vi "Part Config.vi"(0 "Loaded Config":T2={"DAQ Settings"={"Trigger Type"=enum."Manual", "Trigger Samples"=0, "Pretrigger Samples"=0, "Trigger Interval"=0.0, "Time Units"=FALSE, "Auto Save"=FALSE, "Sample Rate"=7.0, "Select Analog"=FALSE, "Trigger Value"=0.0, "Trigger Stop Method"=enum."Use Samples Value to Stop Trigger", "Rate Sec/Min"=FALSE, "Save Mode"=enum."Single File", "File Size Limit"=0.0, "Log File Type"=enum."Basic", "Trigger Data Index"=0}, "Channels"=[], "Header"={"TA Number"="", "Test Name"="", "Serial Number"="", "Technician"=""}, "Graph Settings"={"Graph Labels"=[], [], [], [], [], [], [], [], [], [], [], [], [], "Graph Toggles"=[], "Axis Toggles"=[], "Graph Range"=enum."1"}, "Test Limits"=[], "All Type Info"=[], "Save Mode"=enum."Single File"} {"DAQ Settings"."Trigger Interval" min=0.0; "DAQ Settings"."Pretrigger Samples" min=0; "DAQ Settings"."Trigger Samples" min=0}) -> (4 "Config Out":T2={"DAQ Settings"={"Trigger Type"=enum."Manual", "Trigger Samples"=0, "Pretrigger Samples"=0, "Trigger Interval"=0.0, "Time Units"=FALSE, "Auto Save"=FALSE, "Sample Rate"=7.0, "Select Analog"=FALSE, "Trigger Value"=0.0, "Trigger Stop Method"=enum."Use Samples Value to Stop Trigger", "Rate Sec/Min"=FALSE, "Save Mode"=enum."Single File", "File Size Limit"=0.0, "Log File Type"=enum."Basic", "Trigger Data Index"=0}, "Channels"=[], "Header"={"TA Number"="", "Test Name"="", "Serial Number"="", "Technician"=""}, "Graph Settings"={"Graph Labels"=[], [], [], [], [], [], [], [], [], [], [], [], [], "Graph Toggles"=[], "Axis Toggles"=[], "Graph Range"=enum."1"}, "Test Limits"=[], "All Type Info"=[], "Save Mode"=enum."Single File"} {"DAQ Settings"."Trigger Interval" min=0.0; "DAQ Settings"."Pretrigger Samples" min=0; "DAQ Settings"."Trigger Samples" min=0}, 8 "Changes?":bool)   [LabVIEW 2019]
uses:
  Type Defs and Controls/Sensor Config.ctl
  Type Defs and Controls/DAQ Settings.ctl
  Type Defs and Controls/Trigger Stop Method.ctl
  Type Defs and Controls/Log File Type.ctl
  Type Defs and Controls/Channel Config.ctl
  Type Defs and Controls/Header.ctl
  Type Defs and Controls/Graph Settings Type Def.ctl
  Type Defs and Controls/Test Limits.ctl
  Type Defs and Controls/All Part Info.ctl
  Type Defs and Controls/Part Info.ctl
panel:
  in  "Rename":bool
  out "Total Channels":string
  in  "Delete Type":bool
  in  "Add New Type":bool
  in  "Type":u16(ring) items=["<NO SELECTION >", "New Type"]
  in  "Tab Control":enum32{"Main", "Limits"}(tab)
  in  "Part Numbers":cluster{"Part Number":string, "Acquire":bool}[](array[cluster])
  in  "Signals  Names":T1(array[cluster])
  in  "# Signals":u16=1 min=1 max=32 step=1
  in  "# Parts":u16=1 min=1 max=32 step=1
  in  "Signal Style":enum16{"Steady State", "Cyclic"}(ring)
  out "Current Limit Selection:":string
  in  "RMS Minimum":dbl format="%.3f "
  in  "RMS Maximum":dbl format="%.3f "
  in  "Enable Limits":bool
  in  "Pk-Pk Minimum":dbl format="%.3f "
  in  "Pk-Pk Maximum":dbl format="%.3f "
  in  "Enable Limits":bool
  in  "EU Low State Min":dbl format="%.3f "
  in  "EU Low State Max":dbl format="%.3f "
  in  "EU High State Min":dbl caption="EU Minimum" format="%.3f "
  in  "EU High State Max":dbl caption="EU Maximum" format="%.3f "
  in  "Freq Minimum":dbl format="%.1f Hz"
  in  "Freq Maximum":dbl format="%.1f Hz"
  in  "Enable Limits":bool
  in  "Cancel":bool
  in  "OK":bool
  # "All Signals that have matching High and Low Limits\nwill not be in Functional data file."
  # "RMS Limits"
  # "EU Limits Type"
  # "Pk-Pk Limits"
  # "Frequency Limits"
  # "All Signals that have matching High and Low Limits will not be in Functional data file."
  # "EGU"
  # "EGU"
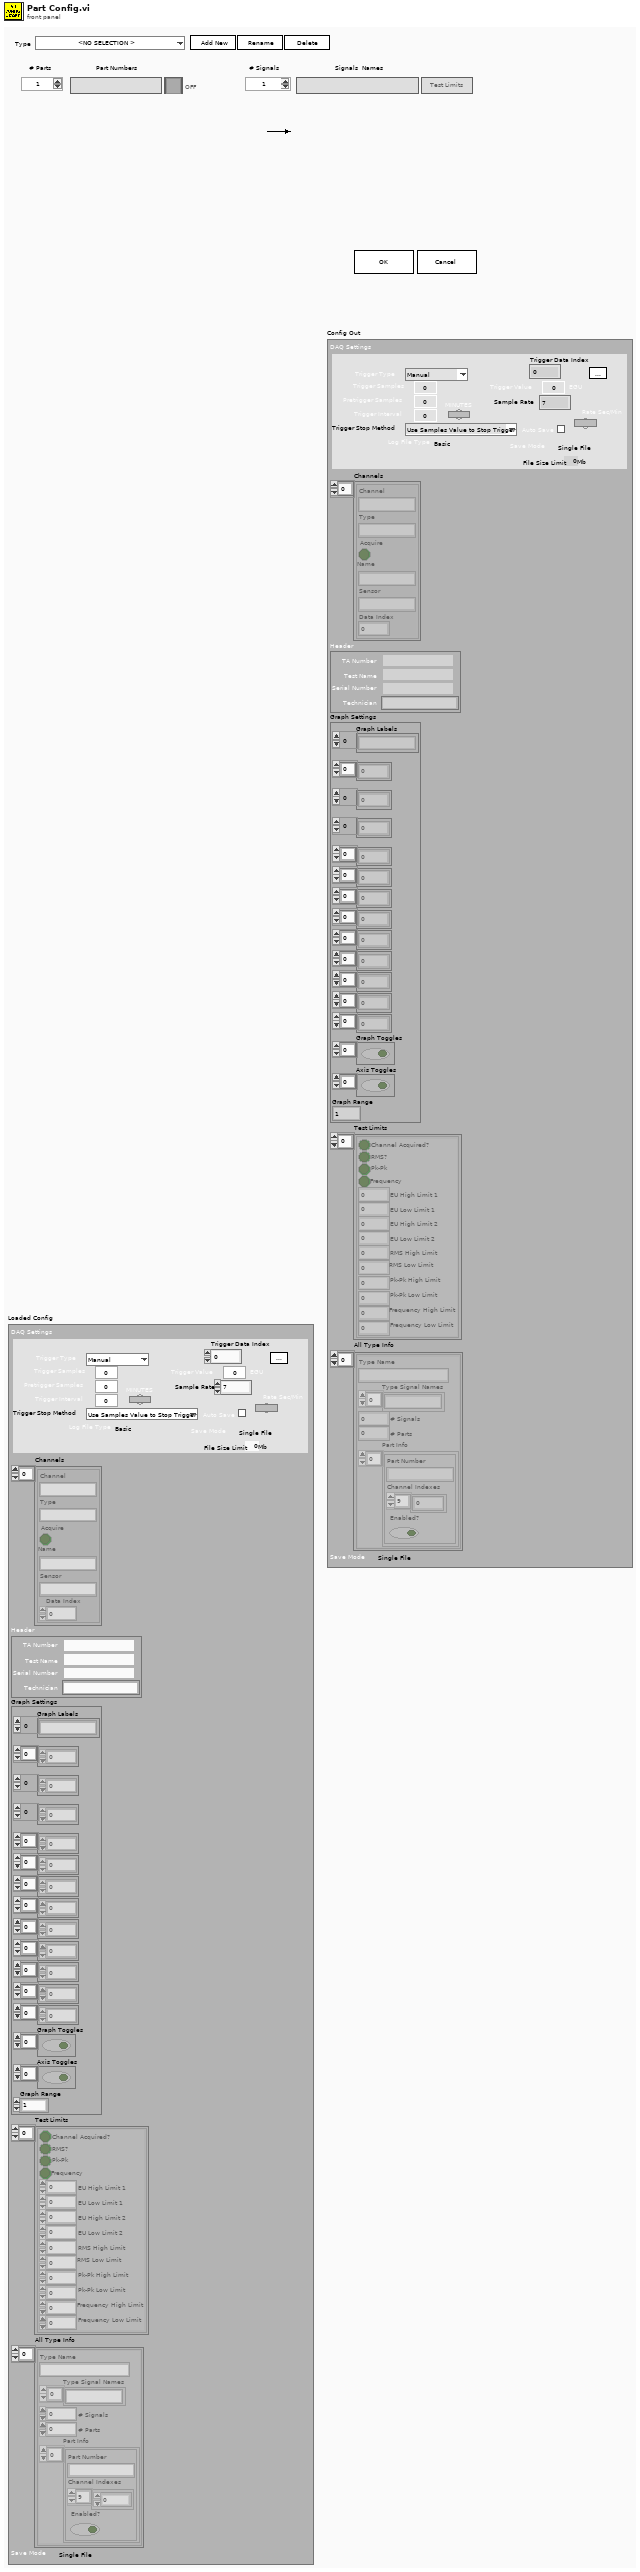
[diagram p1: front panel]
types:
  T1 = cluster{"Signal Names":string, "Test Limits":bool}[]
  T2 = typedef "Sensor Config.ctl" = cluster{"DAQ Settings":T3, "Channels":T6[], "Header":T7, "Graph Settings":T8, "Test Limits":T9[], "All Type Info":T10, "Save Mode":enum16{"Single File", "Segmented Files", "New File at Midnight"}}
  T3 = typedef "DAQ Settings.ctl" = cluster{"Trigger Type":enum16{"Manual", "Timed", "Analog Rising", "Analog Falling"}, "Trigger Samples":i32, "Pretrigger Samples":i32, "Trigger Interval":dbl, "Time Units":bool, "Auto Save":bool, "Sample Rate":dbl, "Select Analog":bool, "Trigger Value":dbl, "Trigger Stop Method":T4, "Rate Sec/Min":bool, "Save Mode":enum16{"Single File", "Segmented Files", "New File at Midnight"}, "File Size Limit":dbl, "Log File Type":T5, "Trigger Data Index":u32}
  T4 = typedef "Trigger Stop Method.ctl" = enum16{"Use Samples Value to Stop Trigger", "Use Threshold to Stop Trigger"}
  T5 = typedef "Log File Type.ctl" = enum16{"Basic", "RTS"}
  T6 = typedef "Channel Config.ctl" = cluster{"Channel":string, "Type":string, "Acquire":bool, "Name":string, "Sensor":string, "Data Index":u32}
  T7 = typedef "Header.ctl" = cluster{"TA Number":string, "Test Name":string, "Serial Number":string, "Technician":string}
  T8 = typedef "Graph Settings Type Def.ctl" = cluster{"Graph Labels":string[], u8[], i16[], u32[], u8[], u8[], u8[], u32[], u8[], u8[], u8[], dbl[], dbl[], "Graph Toggles":bool[], "Axis Toggles":bool[], "Graph Range":enum16{"1", "2", "3", "4", "5", "10", "15", "30", "60"}}
  T9 = typedef "Test Limits.ctl" = cluster{"Channel Acquired?":bool, "RMS?":bool, "Pk-Pk":bool, "Frequency":bool, "EU High Limit 1":dbl, "EU Low Limit 1":dbl, "EU High Limit 2":dbl, "EU Low Limit 2":dbl, "RMS High Limit":dbl, "RMS Low Limit":dbl, "Pk-Pk High Limit ":dbl, "Pk-Pk Low Limit":dbl, "Frequency High Limit":dbl, "Frequency Low Limit":dbl}
  T10 = typedef "All Part Info.ctl" = cluster{"Type Name":string, "Type Signal Names":string[], "# Signals":i32, "# Parts":i32, "Part Info":T11[]}[]
  T11 = typedef "Part Info.ctl" = cluster{"Part Number":string, "Channel Indexes":u16[], "Enabled?":bool}
  T12 = cluster{"Loaded Config":T2, "Modified Config":T2, "Test Limit Index":i32, "Type Index":i32, "All Test Limits":cluster{T9[]}[], "All Type Info":T10, "Last Type Index":i32, "Signal Style Index":i32, "Last Signal Style Index":i32}
  T13 = enum8{"Enabled", "Disabled", "Disabled and Grayed Out"}
  T14 = cluster{"Type Name":string, "Type Signal Names":string[], "# Signals":i32, "# Parts":i32, "Type Info":T11[]}
  T15 = cluster{"Type Name":string, "Type Signal Names":string[], "# Signals":i32, "# Parts":i32, "Part Info":T11[]}
  T16 = cluster{"Type Name":string, "Type Signal Names":string[], "Signals":i32, "# Parts":i32, "Type Info":T11[]}[]
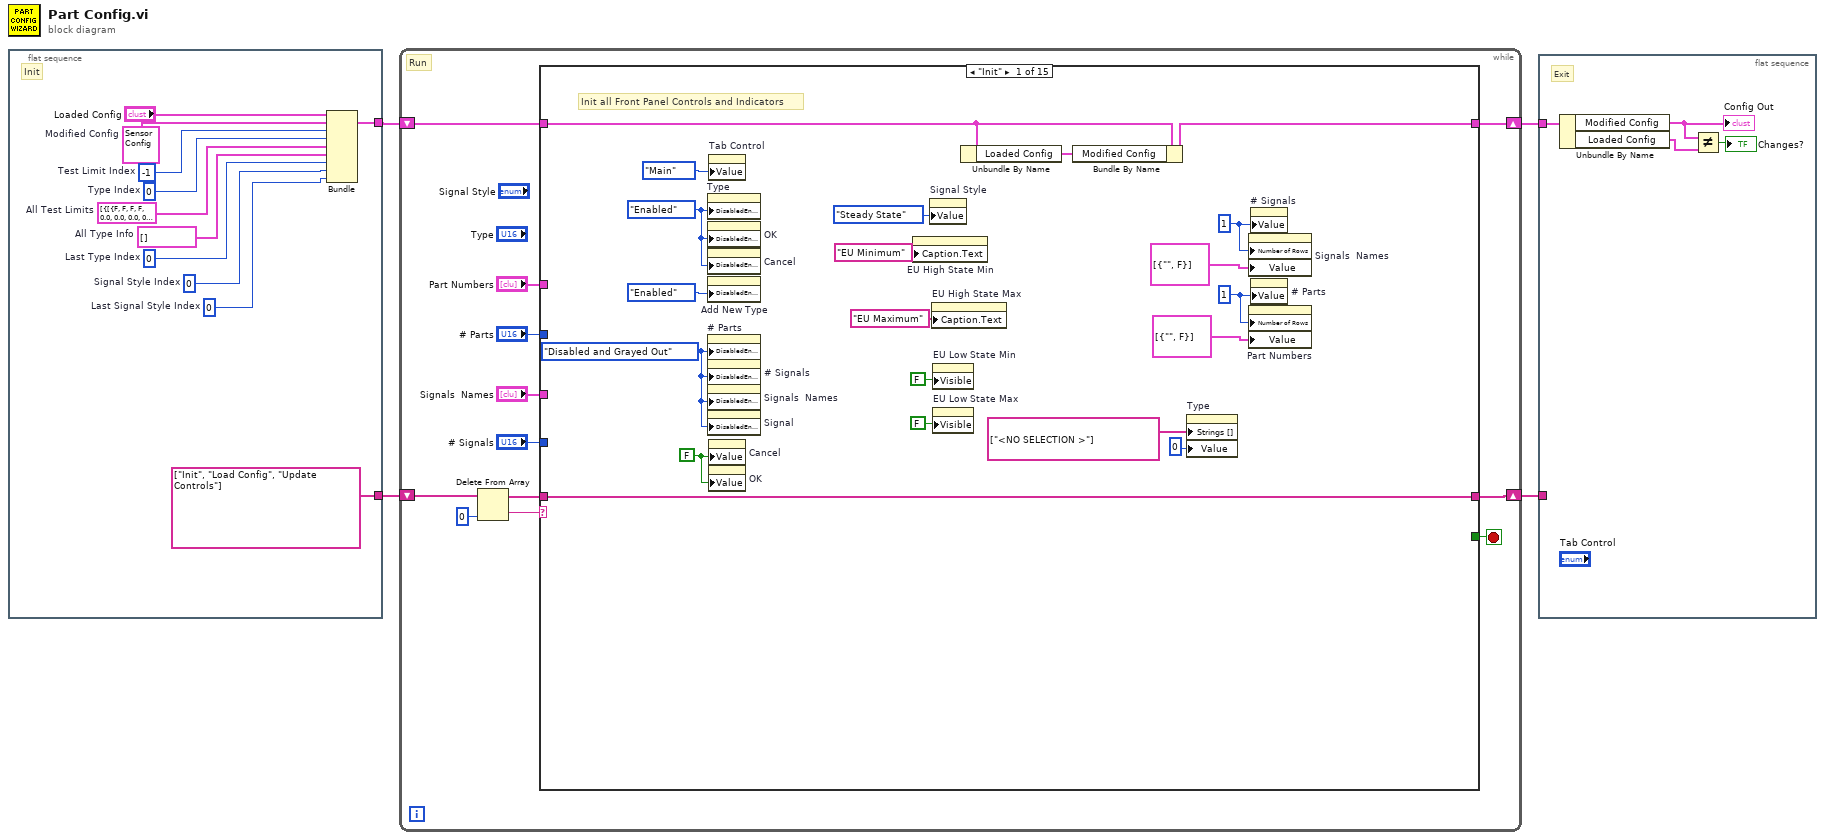
[diagram p0: block diagram]
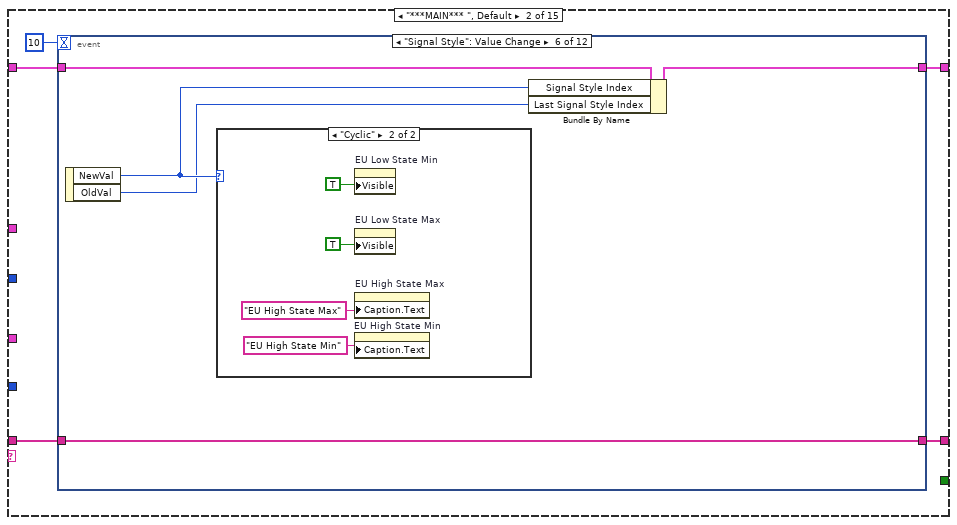
[diagram p2: hidden frame]
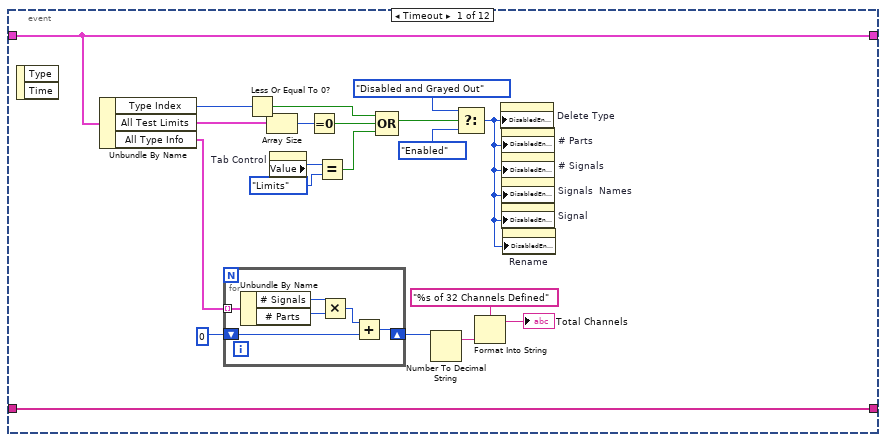
[diagram p3: hidden frame]
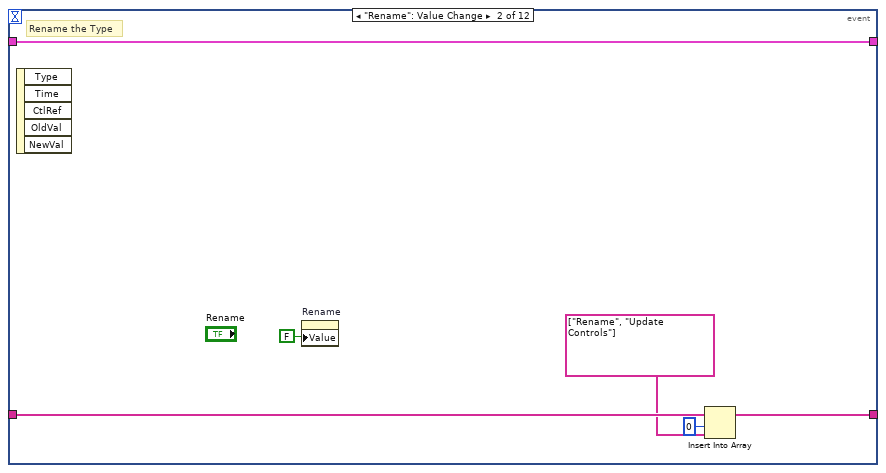
[diagram p4: hidden frame]
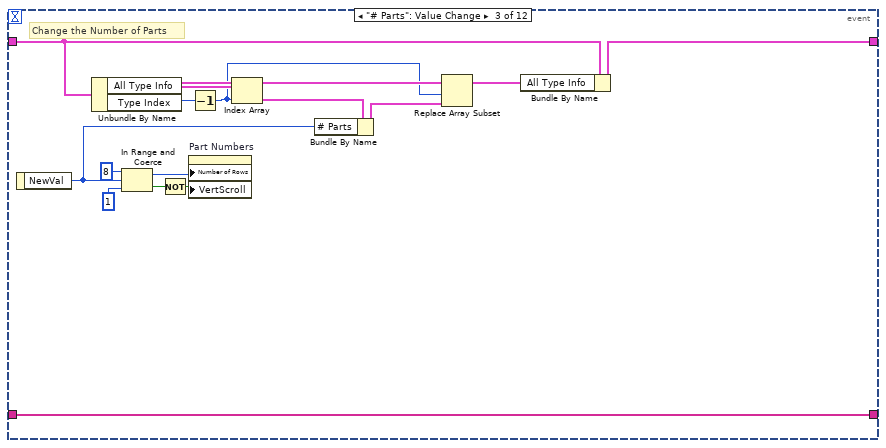
[diagram p5: hidden frame]
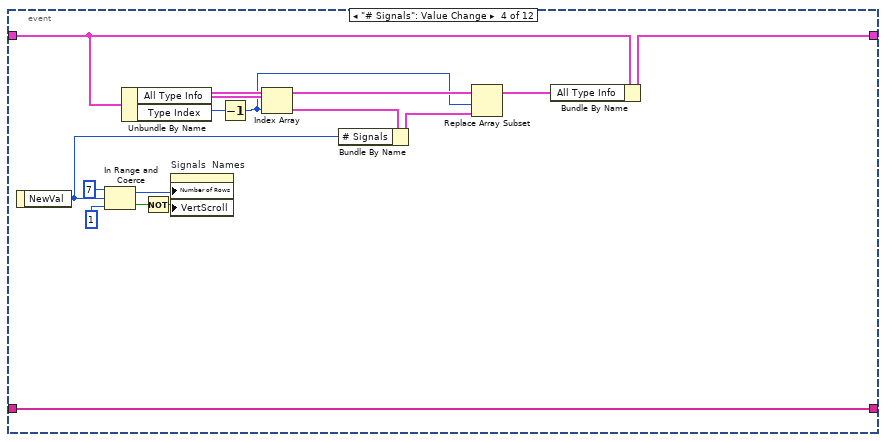
[diagram p6: hidden frame]
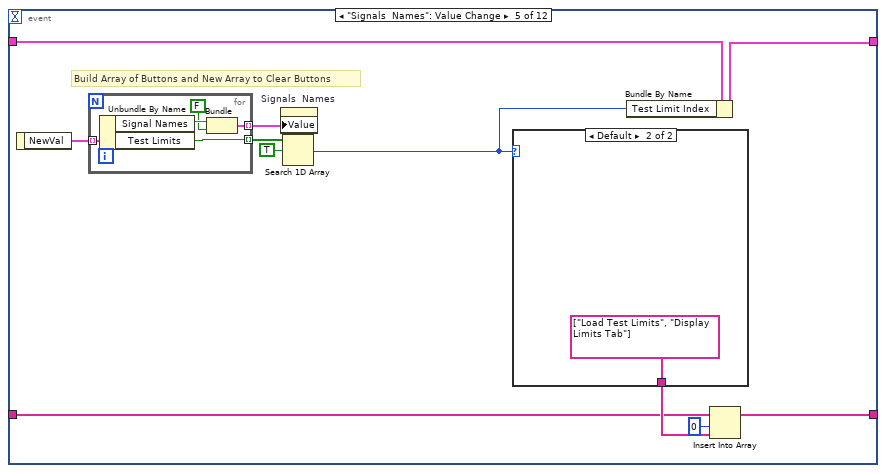
[diagram p7: hidden frame]
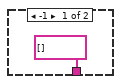
[diagram p8: hidden frame]
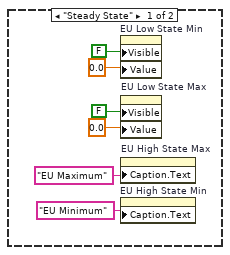
[diagram p9: hidden frame]
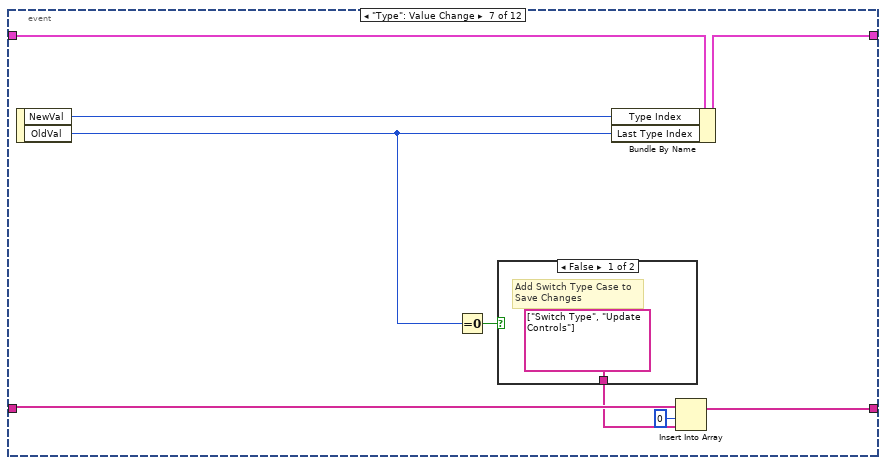
[diagram p10: hidden frame]
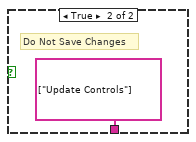
[diagram p11: hidden frame]
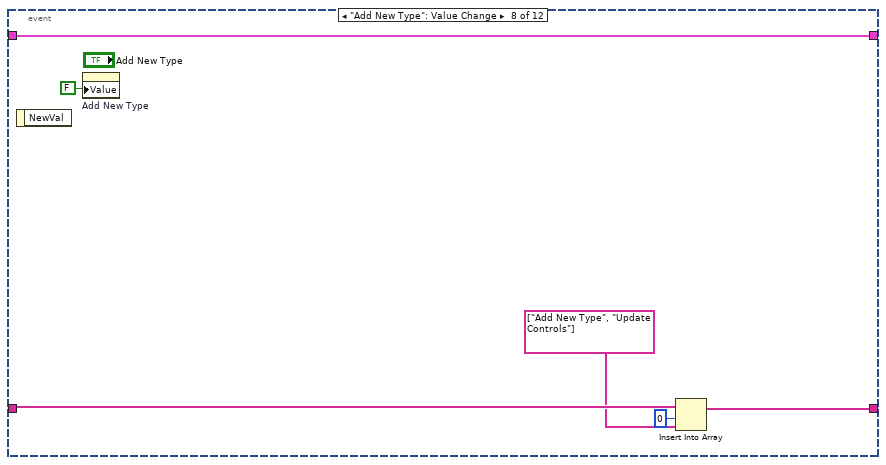
[diagram p12: hidden frame]
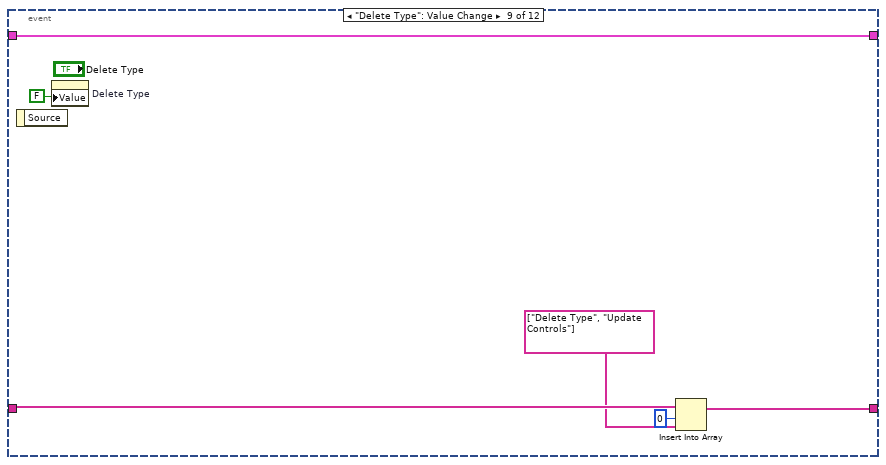
[diagram p13: hidden frame]
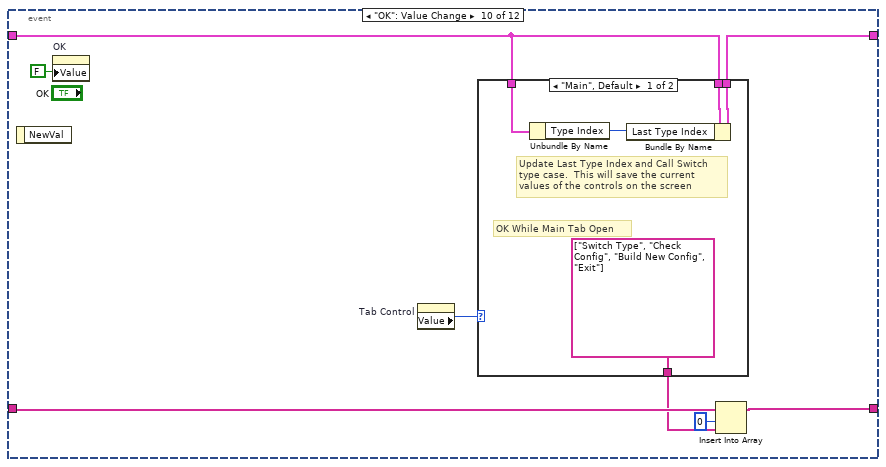
[diagram p14: hidden frame]
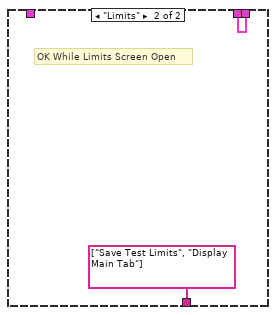
[diagram p15: hidden frame]
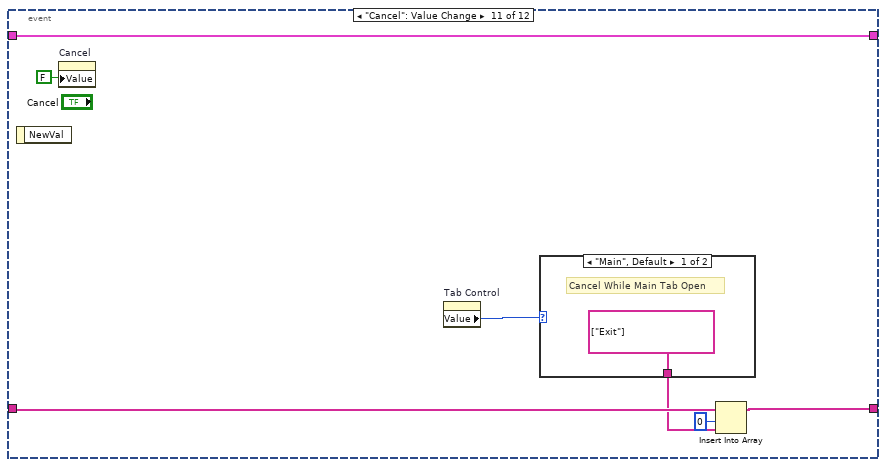
[diagram p16: hidden frame]
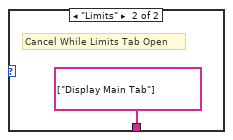
[diagram p17: hidden frame]
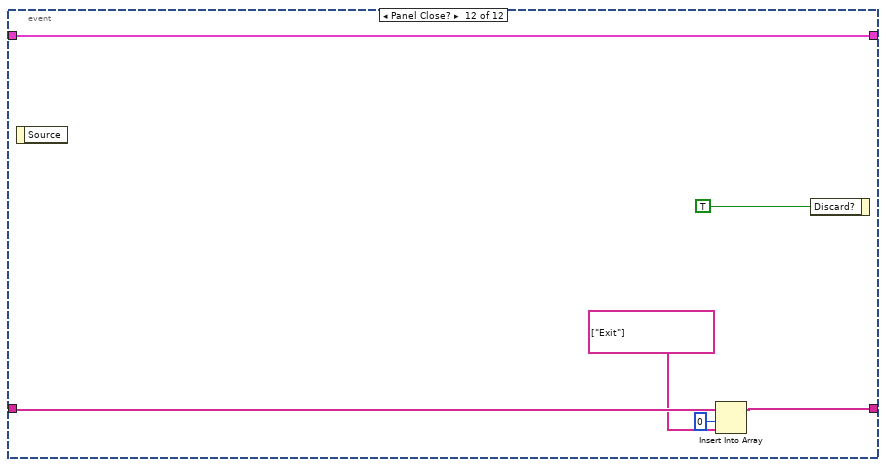
[diagram p18: hidden frame]
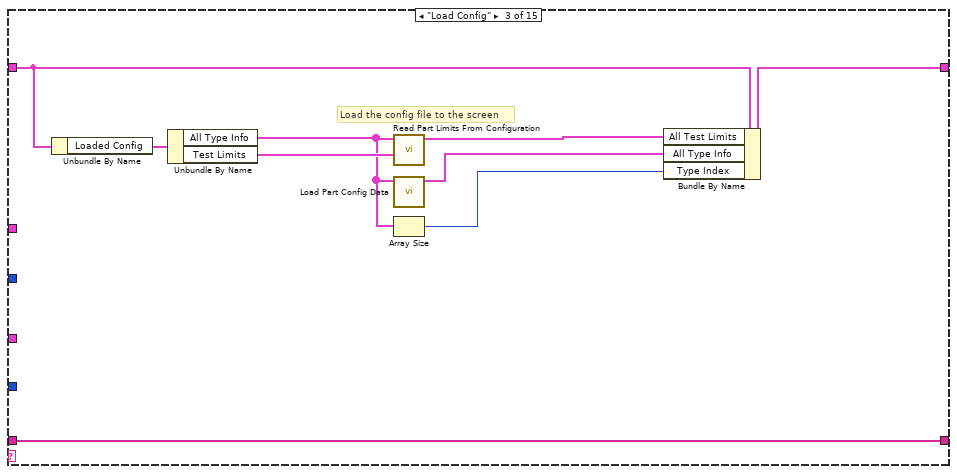
[diagram p19: hidden frame]
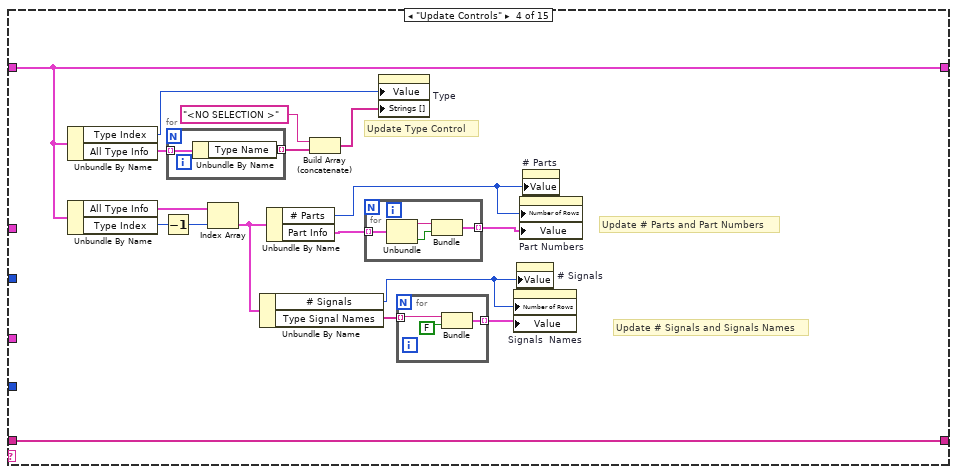
[diagram p20: hidden frame]
diagram:
  n1 = flat-sequence {
    tunnel: [string[] ["Init", "Load Config", "Update Controls"]] -> w4
    tunnel: [w14] -> w3
    frame #0 {
      w5 = 0  # Last Signal Style Index
      w6 = 0  # Signal Style Index
      w7 = 0  # Last Type Index
      w8 = T10 []  # All Type Info
      w9 = cluster{T9[]}[] [{[{"Channel Acquired?"=FALSE, "RMS?"=FALSE, "Pk-Pk"=FALSE, "Frequency"=FALSE, "EU High Limit 1"=0.0, "EU Low Limit 1"=0.0, "EU High Limit 2"=0.0, "EU Low Limit 2"=0.0, "RMS High Limit"=0.0, "RMS Low Limit"=0.0, "Pk-Pk High Limit "=0.0, "Pk-Pk Low Limit"=0.0, "Frequency High Limit"=0.0, "Frequency Low Limit"=0.0}]}, {[{"Channel Acquired?"=FALSE, "RMS?"=FALSE, "Pk-Pk"=FALSE, "Frequency"=FALSE, "EU High Limit 1"=0.0, "EU Low Limit 1"=0.0, "EU High Limit 2"=0.0, "EU Low Limit 2"=0.0, "RMS High Limit"=0.0, "RMS Low Limit"=0.0, "Pk-Pk High Limit "=0.0, "Pk-Pk Low Limit"=0.0, "Frequency High Limit"=0.0, "Frequency Low Limit"=0.0}]}, {[{"Channel Acquired?"=FALSE, "RMS?"=FALSE, "Pk-Pk"=FALSE, "Frequency"=FALSE, "EU High Limit 1"=0.0, "EU Low Limit 1"=0.0, "EU High Limit 2"=0.0, "EU Low Limit 2"=0.0, "RMS High Limit"=0.0, "RMS Low Limit"=0.0, "Pk-Pk High Limit "=0.0, "Pk-Pk Low Limit"=0.0, "Frequency High Limit"=0.0, "Frequency Low Limit"=0.0}]}, {[{"Channel Acquired?"=FALSE, "RMS?"=FALSE, "Pk-Pk"=FALSE, "Frequency"=FALSE, "EU High Limit 1"=0.0, "EU Low Limit 1"=0.0, "EU High Limit 2"=0.0, "EU Low Limit 2"=0.0, "RMS High Limit"=0.0, "RMS Low Limit"=0.0, "Pk-Pk High Limit "=0.0, "Pk-Pk Low Limit"=0.0, "Frequency High Limit"=0.0, "Frequency Low Limit"=0.0}]}, {[{"Channel Acquired?"=FALSE, "RMS?"=FALSE, "Pk-Pk"=FALSE, "Frequency"=FALSE, "EU High Limit 1"=0.0, "EU Low Limit 1"=0.0, "EU High Limit 2"=0.0, "EU Low Limit 2"=0.0, "RMS High Limit"=0.0, "RMS Low Limit"=0.0, "Pk-Pk High Limit "=0.0, "Pk-Pk Low Limit"=0.0, "Frequency High Limit"=0.0, "Frequency Low Limit"=0.0}]}, {[{"Channel Acquired?"=FALSE, "RMS?"=FALSE, "Pk-Pk"=FALSE, "Frequency"=FALSE, "EU High Limit 1"=0.0, "EU Low Limit 1"=0.0, "EU High Limit 2"=0.0, "EU Low Limit 2"=0.0, "RMS High Limit"=0.0, "RMS Low Limit"=0.0, "Pk-Pk High Limit "=0.0, "Pk-Pk Low Limit"=0.0, "Frequency High Limit"=0.0, "Frequency Low Limit"=0.0}]}, {[{"Channel Acquired?"=FALSE, "RMS?"=FALSE, "Pk-Pk"=FALSE, "Frequency"=FALSE, "EU High Limit 1"=0.0, "EU Low Limit 1"=0.0, "EU High Limit 2"=0.0, "EU Low Limit 2"=0.0, "RMS High Limit"=0.0, "RMS Low Limit"=0.0, "Pk-Pk High Limit "=0.0, "Pk-Pk Low Limit"=0.0, "Frequency High Limit"=0.0, "Frequency Low Limit"=0.0}]}, {[{"Channel Acquired?"=FALSE, "RMS?"=FALSE, "Pk-Pk"=FALSE, "Frequency"=FALSE, "EU High Limit 1"=0.0, "EU Low Limit 1"=0.0, "EU High Limit 2"=0.0, "EU Low Limit 2"=0.0, "RMS High Limit"=0.0, "RMS Low Limit"=0.0, "Pk-Pk High Limit "=0.0, "Pk-Pk Low Limit"=0.0, "Frequency High Limit"=0.0, "Frequency Low Limit"=0.0}]}, {[{"Channel Acquired?"=FALSE, "RMS?"=FALSE, "Pk-Pk"=FALSE, "Frequency"=FALSE, "EU High Limit 1"=0.0, "EU Low Limit 1"=0.0, "EU High Limit 2"=0.0, "EU Low Limit 2"=0.0, "RMS High Limit"=0.0, "RMS Low Limit"=0.0, "Pk-Pk High Limit "=0.0, "Pk-Pk Low Limit"=0.0, "Frequency High Limit"=0.0, "Frequency Low Limit"=0.0}]}, {[{"Channel Acquired?"=FALSE, "RMS?"=FALSE, "Pk-Pk"=FALSE, "Frequency"=FALSE, "EU High Limit 1"=0.0, "EU Low Limit 1"=0.0, "EU High Limit 2"=0.0, "EU Low Limit 2"=0.0, "RMS High Limit"=0.0, "RMS Low Limit"=0.0, "Pk-Pk High Limit "=0.0, "Pk-Pk Low Limit"=0.0, "Frequency High Limit"=0.0, "Frequency Low Limit"=0.0}]}, {[{"Channel Acquired?"=FALSE, "RMS?"=FALSE, "Pk-Pk"=FALSE, "Frequency"=FALSE, "EU High Limit 1"=0.0, "EU Low Limit 1"=0.0, "EU High Limit 2"=0.0, "EU Low Limit 2"=0.0, "RMS High Limit"=0.0, "RMS Low Limit"=0.0, "Pk-Pk High Limit "=0.0, "Pk-Pk Low Limit"=0.0, "Frequency High Limit"=0.0, "Frequency Low Limit"=0.0}]}, {[{"Channel Acquired?"=FALSE, "RMS?"=FALSE, "Pk-Pk"=FALSE, "Frequency"=FALSE, "EU High Limit 1"=0.0, "EU Low Limit 1"=0.0, "EU High Limit 2"=0.0, "EU Low Limit 2"=0.0, "RMS High Limit"=0.0, "RMS Low Limit"=0.0, "Pk-Pk High Limit "=0.0, "Pk-Pk Low Limit"=0.0, "Frequency High Limit"=0.0, "Frequency Low Limit"=0.0}]}, {[{"Channel Acquired?"=FALSE, "RMS?"=FALSE, "Pk-Pk"=FALSE, "Frequency"=FALSE, "EU High Limit 1"=0.0, "EU Low Limit 1"=0.0, "EU High Limit 2"=0.0, "EU Low Limit 2"=0.0, "RMS High Limit"=0.0, "RMS Low Limit"=0.0, "Pk-Pk High Limit "=0.0, "Pk-Pk Low Limit"=0.0, "Frequency High Limit"=0.0, "Frequency Low Limit"=0.0}]}, {[{"Channel Acquired?"=FALSE, "RMS?"=FALSE, "Pk-Pk"=FALSE, "Frequency"=FALSE, "EU High Limit 1"=0.0, "EU Low Limit 1"=0.0, "EU High Limit 2"=0.0, "EU Low Limit 2"=0.0, "RMS High Limit"=0.0, "RMS Low Limit"=0.0, "Pk-Pk High Limit "=0.0, "Pk-Pk Low Limit"=0.0, "Frequency High Limit"=0.0, "Frequency Low Limit"=0.0}]}, {[{"Channel Acquired?"=FALSE, "RMS?"=FALSE, "Pk-Pk"=FALSE, "Frequency"=FALSE, "EU High Limit 1"=0.0, "EU Low Limit 1"=0.0, "EU High Limit 2"=0.0, "EU Low Limit 2"=0.0, "RMS High Limit"=0.0, "RMS Low Limit"=0.0, "Pk-Pk High Limit "=0.0, "Pk-Pk Low Limit"=0.0, "Frequency High Limit"=0.0, "Frequency Low Limit"=0.0}]}, {[{"Channel Acquired?"=FALSE, "RMS?"=FALSE, "Pk-Pk"=FALSE, "Frequency"=FALSE, "EU High Limit 1"=0.0, "EU Low Limit 1"=0.0, "EU High Limit 2"=0.0, "EU Low Limit 2"=0.0, "RMS High Limit"=0.0, "RMS Low Limit"=0.0, "Pk-Pk High Limit "=0.0, "Pk-Pk Low Limit"=0.0, "Frequency High Limit"=0.0, "Frequency Low Limit"=0.0}]}, {[{"Channel Acquired?"=FALSE, "RMS?"=FALSE, "Pk-Pk"=FALSE, "Frequency"=FALSE, "EU High Limit 1"=0.0, "EU Low Limit 1"=0.0, "EU High Limit 2"=0.0, "EU Low Limit 2"=0.0, "RMS High Limit"=0.0, "RMS Low Limit"=0.0, "Pk-Pk High Limit "=0.0, "Pk-Pk Low Limit"=0.0, "Frequency High Limit"=0.0, "Frequency Low Limit"=0.0}]}, {[{"Channel Acquired?"=FALSE, "RMS?"=FALSE, "Pk-Pk"=FALSE, "Frequency"=FALSE, "EU High Limit 1"=0.0, "EU Low Limit 1"=0.0, "EU High Limit 2"=0.0, "EU Low Limit 2"=0.0, "RMS High Limit"=0.0, "RMS Low Limit"=0.0, "Pk-Pk High Limit "=0.0, "Pk-Pk Low Limit"=0.0, "Frequency High Limit"=0.0, "Frequency Low Limit"=0.0}]}, {[{"Channel Acquired?"=FALSE, "RMS?"=FALSE, "Pk-Pk"=FALSE, "Frequency"=FALSE, "EU High Limit 1"=0.0, "EU Low Limit 1"=0.0, "EU High Limit 2"=0.0, "EU Low Limit 2"=0.0, "RMS High Limit"=0.0, "RMS Low Limit"=0.0, "Pk-Pk High Limit "=0.0, "Pk-Pk Low Limit"=0.0, "Frequency High Limit"=0.0, "Frequency Low Limit"=0.0}]}, {[{"Channel Acquired?"=FALSE, "RMS?"=FALSE, "Pk-Pk"=FALSE, "Frequency"=FALSE, "EU High Limit 1"=0.0, "EU Low Limit 1"=0.0, "EU High Limit 2"=0.0, "EU Low Limit 2"=0.0, "RMS High Limit"=0.0, "RMS Low Limit"=0.0, "Pk-Pk High Limit "=0.0, "Pk-Pk Low Limit"=0.0, "Frequency High Limit"=0.0, "Frequency Low Limit"=0.0}]}, {[{"Channel Acquired?"=FALSE, "RMS?"=FALSE, "Pk-Pk"=FALSE, "Frequency"=FALSE, "EU High Limit 1"=0.0, "EU Low Limit 1"=0.0, "EU High Limit 2"=0.0, "EU Low Limit 2"=0.0, "RMS High Limit"=0.0, "RMS Low Limit"=0.0, "Pk-Pk High Limit "=0.0, "Pk-Pk Low Limit"=0.0, "Frequency High Limit"=0.0, "Frequency Low Limit"=0.0}]}, {[{"Channel Acquired?"=FALSE, "RMS?"=FALSE, "Pk-Pk"=FALSE, "Frequency"=FALSE, "EU High Limit 1"=0.0, "EU Low Limit 1"=0.0, "EU High Limit 2"=0.0, "EU Low Limit 2"=0.0, "RMS High Limit"=0.0, "RMS Low Limit"=0.0, "Pk-Pk High Limit "=0.0, "Pk-Pk Low Limit"=0.0, "Frequency High Limit"=0.0, "Frequency Low Limit"=0.0}]}, {[{"Channel Acquired?"=FALSE, "RMS?"=FALSE, "Pk-Pk"=FALSE, "Frequency"=FALSE, "EU High Limit 1"=0.0, "EU Low Limit 1"=0.0, "EU High Limit 2"=0.0, "EU Low Limit 2"=0.0, "RMS High Limit"=0.0, "RMS Low Limit"=0.0, "Pk-Pk High Limit "=0.0, "Pk-Pk Low Limit"=0.0, "Frequency High Limit"=0.0, "Frequency Low Limit"=0.0}]}, {[{"Channel Acquired?"=FALSE, "RMS?"=FALSE, "Pk-Pk"=FALSE, "Frequency"=FALSE, "EU High Limit 1"=0.0, "EU Low Limit 1"=0.0, "EU High Limit 2"=0.0, "EU Low Limit 2"=0.0, "RMS High Limit"=0.0, "RMS Low Limit"=0.0, "Pk-Pk High Limit "=0.0, "Pk-Pk Low Limit"=0.0, "Frequency High Limit"=0.0, "Frequency Low Limit"=0.0}]}, {[{"Channel Acquired?"=FALSE, "RMS?"=FALSE, "Pk-Pk"=FALSE, "Frequency"=FALSE, "EU High Limit 1"=0.0, "EU Low Limit 1"=0.0, "EU High Limit 2"=0.0, "EU Low Limit 2"=0.0, "RMS High Limit"=0.0, "RMS Low Limit"=0.0, "Pk-Pk High Limit "=0.0, "Pk-Pk Low Limit"=0.0, "Frequency High Limit"=0.0, "Frequency Low Limit"=0.0}]}, {[{"Channel Acquired?"=FALSE, "RMS?"=FALSE, "Pk-Pk"=FALSE, "Frequency"=FALSE, "EU High Limit 1"=0.0, "EU Low Limit 1"=0.0, "EU High Limit 2"=0.0, "EU Low Limit 2"=0.0, "RMS High Limit"=0.0, "RMS Low Limit"=0.0, "Pk-Pk High Limit "=0.0, "Pk-Pk Low Limit"=0.0, "Frequency High Limit"=0.0, "Frequency Low Limit"=0.0}]}, {[{"Channel Acquired?"=FALSE, "RMS?"=FALSE, "Pk-Pk"=FALSE, "Frequency"=FALSE, "EU High Limit 1"=0.0, "EU Low Limit 1"=0.0, "EU High Limit 2"=0.0, "EU Low Limit 2"=0.0, "RMS High Limit"=0.0, "RMS Low Limit"=0.0, "Pk-Pk High Limit "=0.0, "Pk-Pk Low Limit"=0.0, "Frequency High Limit"=0.0, "Frequency Low Limit"=0.0}]}, {[{"Channel Acquired?"=FALSE, "RMS?"=FALSE, "Pk-Pk"=FALSE, "Frequency"=FALSE, "EU High Limit 1"=0.0, "EU Low Limit 1"=0.0, "EU High Limit 2"=0.0, "EU Low Limit 2"=0.0, "RMS High Limit"=0.0, "RMS Low Limit"=0.0, "Pk-Pk High Limit "=0.0, "Pk-Pk Low Limit"=0.0, "Frequency High Limit"=0.0, "Frequency Low Limit"=0.0}]}, {[{"Channel Acquired?"=FALSE, "RMS?"=FALSE, "Pk-Pk"=FALSE, "Frequency"=FALSE, "EU High Limit 1"=0.0, "EU Low Limit 1"=0.0, "EU High Limit 2"=0.0, "EU Low Limit 2"=0.0, "RMS High Limit"=0.0, "RMS Low Limit"=0.0, "Pk-Pk High Limit "=0.0, "Pk-Pk Low Limit"=0.0, "Frequency High Limit"=0.0, "Frequency Low Limit"=0.0}]}, {[{"Channel Acquired?"=FALSE, "RMS?"=FALSE, "Pk-Pk"=FALSE, "Frequency"=FALSE, "EU High Limit 1"=0.0, "EU Low Limit 1"=0.0, "EU High Limit 2"=0.0, "EU Low Limit 2"=0.0, "RMS High Limit"=0.0, "RMS Low Limit"=0.0, "Pk-Pk High Limit "=0.0, "Pk-Pk Low Limit"=0.0, "Frequency High Limit"=0.0, "Frequency Low Limit"=0.0}]}, {[{"Channel Acquired?"=FALSE, "RMS?"=FALSE, "Pk-Pk"=FALSE, "Frequency"=FALSE, "EU High Limit 1"=0.0, "EU Low Limit 1"=0.0, "EU High Limit 2"=0.0, "EU Low Limit 2"=0.0, "RMS High Limit"=0.0, "RMS Low Limit"=0.0, "Pk-Pk High Limit "=0.0, "Pk-Pk Low Limit"=0.0, "Frequency High Limit"=0.0, "Frequency Low Limit"=0.0}]}, {[{"Channel Acquired?"=FALSE, "RMS?"=FALSE, "Pk-Pk"=FALSE, "Frequency"=FALSE, "EU High Limit 1"=0.0, "EU Low Limit 1"=0.0, "EU High Limit 2"=0.0, "EU Low Limit 2"=0.0, "RMS High Limit"=0.0, "RMS Low Limit"=0.0, "Pk-Pk High Limit "=0.0, "Pk-Pk Low Limit"=0.0, "Frequency High Limit"=0.0, "Frequency Low Limit"=0.0}, {"Channel Acquired?"=FALSE, "RMS?"=FALSE, "Pk-Pk"=FALSE, "Frequency"=FALSE, "EU High Limit 1"=0.0, "EU Low Limit 1"=0.0, "EU High Limit 2"=0.0, "EU Low Limit 2"=0.0, "RMS High Limit"=0.0, "RMS Low Limit"=0.0, "Pk-Pk High Limit "=0.0, "Pk-Pk Low Limit"=0.0, "Frequency High Limit"=0.0, "Frequency Low Limit"=0.0}, {"Channel Acquired?"=FALSE, "RMS?"=FALSE, "Pk-Pk"=FALSE, "Frequency"=FALSE, "EU High Limit 1"=0.0, "EU Low Limit 1"=0.0, "EU High Limit 2"=0.0, "EU Low Limit 2"=0.0, "RMS High Limit"=0.0, "RMS Low Limit"=0.0, "Pk-Pk High Limit "=0.0, "Pk-Pk Low Limit"=0.0, "Frequency High Limit"=0.0, "Frequency Low Limit"=0.0}, {"Channel Acquired?"=FALSE, "RMS?"=FALSE, "Pk-Pk"=FALSE, "Frequency"=FALSE, "EU High Limit 1"=0.0, "EU Low Limit 1"=0.0, "EU High Limit 2"=0.0, "EU Low Limit 2"=0.0, "RMS High Limit"=0.0, "RMS Low Limit"=0.0, "Pk-Pk High Limit "=0.0, "Pk-Pk Low Limit"=0.0, "Frequency High Limit"=0.0, "Frequency Low Limit"=0.0}, {"Channel Acquired?"=FALSE, "RMS?"=FALSE, "Pk-Pk"=FALSE, "Frequency"=FALSE, "EU High Limit 1"=0.0, "EU Low Limit 1"=0.0, "EU High Limit 2"=0.0, "EU Low Limit 2"=0.0, "RMS High Limit"=0.0, "RMS Low Limit"=0.0, "Pk-Pk High Limit "=0.0, "Pk-Pk Low Limit"=0.0, "Frequency High Limit"=0.0, "Frequency Low Limit"=0.0}, {"Channel Acquired?"=FALSE, "RMS?"=FALSE, "Pk-Pk"=FALSE, "Frequency"=FALSE, "EU High Limit 1"=0.0, "EU Low Limit 1"=0.0, "EU High Limit 2"=0.0, "EU Low Limit 2"=0.0, "RMS High Limit"=0.0, "RMS Low Limit"=0.0, "Pk-Pk High Limit "=0.0, "Pk-Pk Low Limit"=0.0, "Frequency High Limit"=0.0, "Frequency Low Limit"=0.0}, {"Channel Acquired?"=FALSE, "RMS?"=FALSE, "Pk-Pk"=FALSE, "Frequency"=FALSE, "EU High Limit 1"=0.0, "EU Low Limit 1"=0.0, "EU High Limit 2"=0.0, "EU Low Limit 2"=0.0, "RMS High Limit"=0.0, "RMS Low Limit"=0.0, "Pk-Pk High Limit "=0.0, "Pk-Pk Low Limit"=0.0, "Frequency High Limit"=0.0, "Frequency Low Limit"=0.0}, {"Channel Acquired?"=FALSE, "RMS?"=FALSE, "Pk-Pk"=FALSE, "Frequency"=FALSE, "EU High Limit 1"=0.0, "EU Low Limit 1"=0.0, "EU High Limit 2"=0.0, "EU Low Limit 2"=0.0, "RMS High Limit"=0.0, "RMS Low Limit"=0.0, "Pk-Pk High Limit "=0.0, "Pk-Pk Low Limit"=0.0, "Frequency High Limit"=0.0, "Frequency Low Limit"=0.0}, {"Channel Acquired?"=FALSE, "RMS?"=FALSE, "Pk-Pk"=FALSE, "Frequency"=FALSE, "EU High Limit 1"=0.0, "EU Low Limit 1"=0.0, "EU High Limit 2"=0.0, "EU Low Limit 2"=0.0, "RMS High Limit"=0.0, "RMS Low Limit"=0.0, "Pk-Pk High Limit "=0.0, "Pk-Pk Low Limit"=0.0, "Frequency High Limit"=0.0, "Frequency Low Limit"=0.0}, {"Channel Acquired?"=FALSE, "RMS?"=FALSE, "Pk-Pk"=FALSE, "Frequency"=FALSE, "EU High Limit 1"=0.0, "EU Low Limit 1"=0.0, "EU High Limit 2"=0.0, "EU Low Limit 2"=0.0, "RMS High Limit"=0.0, "RMS Low Limit"=0.0, "Pk-Pk High Limit "=0.0, "Pk-Pk Low Limit"=0.0, "Frequency High Limit"=0.0, "Frequency Low Limit"=0.0}, {"Channel Acquired?"=FALSE, "RMS?"=FALSE, "Pk-Pk"=FALSE, "Frequency"=FALSE, "EU High Limit 1"=0.0, "EU Low Limit 1"=0.0, "EU High Limit 2"=0.0, "EU Low Limit 2"=0.0, "RMS High Limit"=0.0, "RMS Low Limit"=0.0, "Pk-Pk High Limit "=0.0, "Pk-Pk Low Limit"=0.0, "Frequency High Limit"=0.0, "Frequency Low Limit"=0.0}, {"Channel Acquired?"=FALSE, "RMS?"=FALSE, "Pk-Pk"=FALSE, "Frequency"=FALSE, "EU High Limit 1"=0.0, "EU Low Limit 1"=0.0, "EU High Limit 2"=0.0, "EU Low Limit 2"=0.0, "RMS High Limit"=0.0, "RMS Low Limit"=0.0, "Pk-Pk High Limit "=0.0, "Pk-Pk Low Limit"=0.0, "Frequency High Limit"=0.0, "Frequency Low Limit"=0.0}, {"Channel Acquired?"=FALSE, "RMS?"=FALSE, "Pk-Pk"=FALSE, "Frequency"=FALSE, "EU High Limit 1"=0.0, "EU Low Limit 1"=0.0, "EU High Limit 2"=0.0, "EU Low Limit 2"=0.0, "RMS High Limit"=0.0, "RMS Low Limit"=0.0, "Pk-Pk High Limit "=0.0, "Pk-Pk Low Limit"=0.0, "Frequency High Limit"=0.0, "Frequency Low Limit"=0.0}, {"Channel Acquired?"=FALSE, "RMS?"=FALSE, "Pk-Pk"=FALSE, "Frequency"=FALSE, "EU High Limit 1"=0.0, "EU Low Limit 1"=0.0, "EU High Limit 2"=0.0, "EU Low Limit 2"=0.0, "RMS High Limit"=0.0, "RMS Low Limit"=0.0, "Pk-Pk High Limit "=0.0, "Pk-Pk Low Limit"=0.0, "Frequency High Limit"=0.0, "Frequency Low Limit"=0.0}, {"Channel Acquired?"=FALSE, "RMS?"=FALSE, "Pk-Pk"=FALSE, "Frequency"=FALSE, "EU High Limit 1"=0.0, "EU Low Limit 1"=0.0, "EU High Limit 2"=0.0, "EU Low Limit 2"=0.0, "RMS High Limit"=0.0, "RMS Low Limit"=0.0, "Pk-Pk High Limit "=0.0, "Pk-Pk Low Limit"=0.0, "Frequency High Limit"=0.0, "Frequency Low Limit"=0.0}, {"Channel Acquired?"=FALSE, "RMS?"=FALSE, "Pk-Pk"=FALSE, "Frequency"=FALSE, "EU High Limit 1"=0.0, "EU Low Limit 1"=0.0, "EU High Limit 2"=0.0, "EU Low Limit 2"=0.0, "RMS High Limit"=0.0, "RMS Low Limit"=0.0, "Pk-Pk High Limit "=0.0, "Pk-Pk Low Limit"=0.0, "Frequency High Limit"=0.0, "Frequency Low Limit"=0.0}, {"Channel Acquired?"=FALSE, "RMS?"=FALSE, "Pk-Pk"=FALSE, "Frequency"=FALSE, "EU High Limit 1"=0.0, "EU Low Limit 1"=0.0, "EU High Limit 2"=0.0, "EU Low Limit 2"=0.0, "RMS High Limit"=0.0, "RMS Low Limit"=0.0, "Pk-Pk High Limit "=0.0, "Pk-Pk Low Limit"=0.0, "Frequency High Limit"=0.0, "Frequency Low Limit"=0.0}, {"Channel Acquired?"=FALSE, "RMS?"=FALSE, "Pk-Pk"=FALSE, "Frequency"=FALSE, "EU High Limit 1"=0.0, "EU Low Limit 1"=0.0, "EU High Limit 2"=0.0, "EU Low Limit 2"=0.0, "RMS High Limit"=0.0, "RMS Low Limit"=0.0, "Pk-Pk High Limit "=0.0, "Pk-Pk Low Limit"=0.0, "Frequency High Limit"=0.0, "Frequency Low Limit"=0.0}, {"Channel Acquired?"=FALSE, "RMS?"=FALSE, "Pk-Pk"=FALSE, "Frequency"=FALSE, "EU High Limit 1"=0.0, "EU Low Limit 1"=0.0, "EU High Limit 2"=0.0, "EU Low Limit 2"=0.0, "RMS High Limit"=0.0, "RMS Low Limit"=0.0, "Pk-Pk High Limit "=0.0, "Pk-Pk Low Limit"=0.0, "Frequency High Limit"=0.0, "Frequency Low Limit"=0.0}, {"Channel Acquired?"=FALSE, "RMS?"=FALSE, "Pk-Pk"=FALSE, "Frequency"=FALSE, "EU High Limit 1"=0.0, "EU Low Limit 1"=0.0, "EU High Limit 2"=0.0, "EU Low Limit 2"=0.0, "RMS High Limit"=0.0, "RMS Low Limit"=0.0, "Pk-Pk High Limit "=0.0, "Pk-Pk Low Limit"=0.0, "Frequency High Limit"=0.0, "Frequency Low Limit"=0.0}, {"Channel Acquired?"=FALSE, "RMS?"=FALSE, "Pk-Pk"=FALSE, "Frequency"=FALSE, "EU High Limit 1"=0.0, "EU Low Limit 1"=0.0, "EU High Limit 2"=0.0, "EU Low Limit 2"=0.0, "RMS High Limit"=0.0, "RMS Low Limit"=0.0, "Pk-Pk High Limit "=0.0, "Pk-Pk Low Limit"=0.0, "Frequency High Limit"=0.0, "Frequency Low Limit"=0.0}, {"Channel Acquired?"=FALSE, "RMS?"=FALSE, "Pk-Pk"=FALSE, "Frequency"=FALSE, "EU High Limit 1"=0.0, "EU Low Limit 1"=0.0, "EU High Limit 2"=0.0, "EU Low Limit 2"=0.0, "RMS High Limit"=0.0, "RMS Low Limit"=0.0, "Pk-Pk High Limit "=0.0, "Pk-Pk Low Limit"=0.0, "Frequency High Limit"=0.0, "Frequency Low Limit"=0.0}, {"Channel Acquired?"=FALSE, "RMS?"=FALSE, "Pk-Pk"=FALSE, "Frequency"=FALSE, "EU High Limit 1"=0.0, "EU Low Limit 1"=0.0, "EU High Limit 2"=0.0, "EU Low Limit 2"=0.0, "RMS High Limit"=0.0, "RMS Low Limit"=0.0, "Pk-Pk High Limit "=0.0, "Pk-Pk Low Limit"=0.0, "Frequency High Limit"=0.0, "Frequency Low Limit"=0.0}, {"Channel Acquired?"=FALSE, "RMS?"=FALSE, "Pk-Pk"=FALSE, "Frequency"=FALSE, "EU High Limit 1"=0.0, "EU Low Limit 1"=0.0, "EU High Limit 2"=0.0, "EU Low Limit 2"=0.0, "RMS High Limit"=0.0, "RMS Low Limit"=0.0, "Pk-Pk High Limit "=0.0, "Pk-Pk Low Limit"=0.0, "Frequency High Limit"=0.0, "Frequency Low Limit"=0.0}, {"Channel Acquired?"=FALSE, "RMS?"=FALSE, "Pk-Pk"=FALSE, "Frequency"=FALSE, "EU High Limit 1"=0.0, "EU Low Limit 1"=0.0, "EU High Limit 2"=0.0, "EU Low Limit 2"=0.0, "RMS High Limit"=0.0, "RMS Low Limit"=0.0, "Pk-Pk High Limit "=0.0, "Pk-Pk Low Limit"=0.0, "Frequency High Limit"=0.0, "Frequency Low Limit"=0.0}, {"Channel Acquired?"=FALSE, "RMS?"=FALSE, "Pk-Pk"=FALSE, "Frequency"=FALSE, "EU High Limit 1"=0.0, "EU Low Limit 1"=0.0, "EU High Limit 2"=0.0, "EU Low Limit 2"=0.0, "RMS High Limit"=0.0, "RMS Low Limit"=0.0, "Pk-Pk High Limit "=0.0, "Pk-Pk Low Limit"=0.0, "Frequency High Limit"=0.0, "Frequency Low Limit"=0.0}, {"Channel Acquired?"=FALSE, "RMS?"=FALSE, "Pk-Pk"=FALSE, "Frequency"=FALSE, "EU High Limit 1"=0.0, "EU Low Limit 1"=0.0, "EU High Limit 2"=0.0, "EU Low Limit 2"=0.0, "RMS High Limit"=0.0, "RMS Low Limit"=0.0, "Pk-Pk High Limit "=0.0, "Pk-Pk Low Limit"=0.0, "Frequency High Limit"=0.0, "Frequency Low Limit"=0.0}, {"Channel Acquired?"=FALSE, "RMS?"=FALSE, "Pk-Pk"=FALSE, "Frequency"=FALSE, "EU High Limit 1"=0.0, "EU Low Limit 1"=0.0, "EU High Limit 2"=0.0, "EU Low Limit 2"=0.0, "RMS High Limit"=0.0, "RMS Low Limit"=0.0, "Pk-Pk High Limit "=0.0, "Pk-Pk Low Limit"=0.0, "Frequency High Limit"=0.0, "Frequency Low Limit"=0.0}, {"Channel Acquired?"=FALSE, "RMS?"=FALSE, "Pk-Pk"=FALSE, "Frequency"=FALSE, "EU High Limit 1"=0.0, "EU Low Limit 1"=0.0, "EU High Limit 2"=0.0, "EU Low Limit 2"=0.0, "RMS High Limit"=0.0, "RMS Low Limit"=0.0, "Pk-Pk High Limit "=0.0, "Pk-Pk Low Limit"=0.0, "Frequency High Limit"=0.0, "Frequency Low Limit"=0.0}, {"Channel Acquired?"=FALSE, "RMS?"=FALSE, "Pk-Pk"=FALSE, "Frequency"=FALSE, "EU High Limit 1"=0.0, "EU Low Limit 1"=0.0, "EU High Limit 2"=0.0, "EU Low Limit 2"=0.0, "RMS High Limit"=0.0, "RMS Low Limit"=0.0, "Pk-Pk High Limit "=0.0, "Pk-Pk Low Limit"=0.0, "Frequency High Limit"=0.0, "Frequency Low Limit"=0.0}, {"Channel Acquired?"=FALSE, "RMS?"=FALSE, "Pk-Pk"=FALSE, "Frequency"=FALSE, "EU High Limit 1"=0.0, "EU Low Limit 1"=0.0, "EU High Limit 2"=0.0, "EU Low Limit 2"=0.0, "RMS High Limit"=0.0, "RMS Low Limit"=0.0, "Pk-Pk High Limit "=0.0, "Pk-Pk Low Limit"=0.0, "Frequency High Limit"=0.0, "Frequency Low Limit"=0.0}, {"Channel Acquired?"=FALSE, "RMS?"=FALSE, "Pk-Pk"=FALSE, "Frequency"=FALSE, "EU High Limit 1"=0.0, "EU Low Limit 1"=0.0, "EU High Limit 2"=0.0, "EU Low Limit 2"=0.0, "RMS High Limit"=0.0, "RMS Low Limit"=0.0, "Pk-Pk High Limit "=0.0, "Pk-Pk Low Limit"=0.0, "Frequency High Limit"=0.0, "Frequency Low Limit"=0.0}]}]  # All Test Limits
      w10 = T2 {"DAQ Settings"={"Trigger Type"=enum."Manual", "Trigger Samples"=0, "Pretrigger Samples"=0, "Trigger Interval"=0.0, "Time Units"=FALSE, "Auto Save"=FALSE, "Sample Rate"=0.0, "Select Analog"=FALSE, "Trigger Value"=0.0, "Trigger Stop Method"=enum."Use Samples Value to Stop Trigger", "Rate Sec/Min"=FALSE, "Save Mode"=enum."Single File", "File Size Limit"=0.0, "Log File Type"=enum."Basic", "Trigger Data Index"=0}, "Channels"=[], "Header"={"TA Number"="", "Test Name"="", "Serial Number"="", "Technician"=""}, "Graph Settings"={"Graph Labels"=[], [], [], [], [], [], [], [], [], [], [], [], [], "Graph Toggles"=[], "Axis Toggles"=[], "Graph Range"=enum."1"}, "Test Limits"=[], "All Type Info"=[], "Save Mode"=enum."Single File"}  # Modified Config
      w11 = 0  # Type Index
      w12 = -1  # Test Limit Index
      # "Init"
      n2 = Bundle("Loaded Config"="Loaded Config", "Modified Config"=w10, "Test Limit Index"=w12, "Type Index"=w11, "All Test Limits"=w9, "All Type Info"=w8, "Last Type Index"=w7, "Signal Style Index"=w6, "Last Signal Style Index"=w5) -> (w14:T12)  [unwired: 1 in]
    }
  }
  n3 = while {
    shift-right: [w23] -> w2
    shift-left: w4 -> [w27]
    shift-right: [w20] -> w1
    shift-left: w3 -> [w21]
    stop <- w22 stop-if-true
    # "Run"
    n4 = Delete From Array(array=w27, index=0) -> (deleted portion=w26:string, array with subset deleted=w24:string[])  [unwired: 1 in]
    n5 = case shown="\"Init\"" w26 {
      tunnel: w24 -> [w47 w50 w209 w226 w243 w252 w306 w325 w352 w362 w402 w437 w440 w445 w447]
      tunnel: [w47 w49 w209 w226 w243 w250 w306 w325 w352 w362 w402 w437 w440 w445 w447] -> w23
      tunnel: [_ _ _ _ _ _ _ _ _ _ _ _ _ _ TRUE] -> w22
      tunnel: w21 -> [w35 w52 w206 w210 w239 w257 w297 w319 w350 w357 w401 w413 w441 w446 w448]
      tunnel: [w34 w51 w205 w210 w238 w257 w296 w321 w351 w356 w401 w412 w441 w446 w448] -> w20
      tunnel: "Part Numbers" -> [_ _ _ _ _ _ w303 _ _ _ _ _ _ _ _]
      tunnel: "# Parts" -> [_ _ _ _ _ _ w292 _ _ _ _ _ _ _ _]
      tunnel: "Signals  Names" -> [_ _ _ _ _ _ w294 _ _ _ w386 _ _ _ _]
      tunnel: "# Signals" -> [_ _ _ _ _ _ w291 _ _ _ _ _ _ _ _]
      frame "Init" {
        w39 = u16 1 ("Signals / Part")
        w38 = u16 1 ("# Parts")
        w41 = T13."Disabled and Grayed Out" ("Disabled")
        w44 = FALSE ("Cancel")
        w45 = T13."Enabled" ("Disabled")
        # "Init all Front Panel Controls and Indicators"
        n6 = property on="Type" class="Ring (strict)"("DisabledEnum"=w45) -> ()  [unwired: 2 in, 2 out]
        n7 = property on="OK" class="Bool (strict)"("DisabledEnum"=w45) -> ()  [unwired: 2 in, 2 out]
        n8 = property on="Cancel" class="Bool (strict)"("DisabledEnum"=w45) -> ()  [unwired: 2 in, 2 out]
        n9 = property on="Add New Type" class="Bool (strict)"("DisabledEnum"=T13."Enabled" ("Disabled")) -> ()  [unwired: 2 in, 2 out]
        n10 = property on="# Parts" class="DigNum (strict)"("DisabledEnum"=w41) -> ()  [unwired: 2 in, 2 out]
        n11 = property on="# Signals" class="DigNum (strict)"("DisabledEnum"=w41) -> ()  [unwired: 2 in, 2 out]
        n12 = property on="Signals  Names" class="Arr (strict)"("DisabledEnum"=w41) -> ()  [unwired: 2 in, 2 out]
        n13 = property on="Signal" class="Clust (strict)"("DisabledEnum"=w41) -> ()  [unwired: 2 in, 2 out]
        n14 = property on="Tab Control" class="TabCtl (strict)"("Value"=enum32{"Main", "Limits"}."Main" ("Tab Control")) -> ()  [unwired: 2 in, 2 out]
        n15 = property on="Cancel" class="Bool (strict)"("Value"=w44) -> ()  [unwired: 2 in, 2 out]
        n16 = property on="OK" class="Bool (strict)"("Value"=w44) -> ()  [unwired: 2 in, 2 out]
        n17 = property on="EU High State Min" class="DigNum (strict)"("Caption.Text"="EU Minimum") -> ()  [unwired: 2 in, 2 out]
        n18 = property on="Signal Style" class="Enum (strict)"("Value"=enum16{"Steady State", "Cyclic"}."Steady State" ("Signal Style")) -> ()  [unwired: 2 in, 2 out]
        n19 = property on="EU High State Max" class="DigNum (strict)"("Caption.Text"="EU Maximum") -> ()  [unwired: 2 in, 2 out]
        n20 = property on="EU Low State Min" class="DigNum (strict)"("Visible"=FALSE) -> ()  [unwired: 2 in, 2 out]
        n21 = property on="EU Low State Max" class="DigNum (strict)"("Visible"=FALSE) -> ()  [unwired: 2 in, 2 out]
        n22 = Unbundle By Name(w35) -> ("Loaded Config"=w33:T2)
        n23 = Bundle By Name(cluster=w35, "Modified Config"=w33) -> (w34:T12)
        n24 = property on="Type" class="Ring (strict)"("Strings []"=string[] ["<NO SELECTION >"], "Value"=0) -> ()  [unwired: 2 in, 2 out]
        n25 = property on="Signals  Names" class="Arr (strict)"("Number of Rows"=w39, "Value"=T1 [{"Signal Names"="", "Test Limits"=FALSE}] ("Signals  Names")) -> ()  [unwired: 2 in, 2 out]
        n26 = property on="Part Numbers" class="Arr (strict)"("Number of Rows"=w38, "Value"=cluster{"Part Number":string, "Acquire":bool}[] [{"Part Number"="", "Acquire"=FALSE}] ("Part Numbers")) -> ()  [unwired: 2 in, 2 out]
        n27 = property on="# Signals" class="DigNum (strict)"("Value"=w39) -> ()  [unwired: 2 in, 2 out]
        n28 = property on="# Parts" class="DigNum (strict)"("Value"=w38) -> ()  [unwired: 2 in, 2 out]
      }
      frame "***MAIN*** ", Default {
        n29 = event shown="[5] \"Signal Style\": Value Change" {
          selector: _ -> [_ _ _ _ _ _ _ _ _ _ _ _]
          dyn-events: _ -> [_ _ _ _ _ _ _ _ _ _ _ _]
          timeout: 10 -> [_ _ _ _ _ _ _ _ _ _ _ _]
          tunnel: w52 -> [w71 w80 w89 w101 w117 w136 w152 w160 w166 w171 w192 w200]
          tunnel: [w71 w80 w88 w102 w116 w135 w151 w160 w166 w172 w192 w200] -> w51
          tunnel: w50 -> [w72 w82 w85 w109 w119 w134 w155 w163 w169 w178 w191 w199]
          tunnel: [w72 w83 w85 w109 w118 w134 w156 w164 w170 w177 w190 w198] -> w49
          event Timeout {
            n30 = event-data() -> ()  [unwired: 1 in, 2 out]
            n31 = Unbundle By Name(w71) -> ("Type Index"=w70:i32, "All Test Limits"=w69:cluster{T9[]}[], "All Type Info"=w59:T10)
            n32 = for {
              tunnel: w59 -> [w78] mode=indexing
              shift-right: [w76] -> w54
              shift-left: 0 ("# Signals") -> [w77]
              n33 = Unbundle By Name(w78) -> ("# Signals"=w75:i32, "# Parts"=w74:i32)
              n34 = Multiply(x=w75, y=w74) -> (x*y=w73:i32)
              n35 = Add(x=w73, y=w77) -> (x+y=w76:i32)
            }
            n36 = Less Or Equal To 0?(x=w70) -> (x <= 0?=w66:bool)
            n37 = Array Size(array=w69) -> (size(s)=w68:i32)
            n38 = property on="Tab Control" class="TabCtl (strict)"() -> ("Value"=w62:enum32{"Main", "Limits"})  [unwired: 2 in, 2 out]
            n39 = Equal To 0?(x=w68) -> (x = 0?=w67:bool)
            n40 = Equal?(x=w62, y=enum32{"Main", "Limits"}."Limits") -> (x = y?=w60:bool)
            n41 = Compound Arithmetic op=OR(w66, w67, w60) -> (w65:bool)
            n42 = Number To Decimal String(number=w54) -> (decimal integer string=w57:string)  [unwired: 1 in]
            n43 = Select(t=T13."Disabled and Grayed Out" ("Disabled"), s=w65, f=T13."Enabled" ("Disabled")) -> (s? t:f=w53:T13)
            n44 = Format Into String(format string="%s of 32 Channels Defined", w57) -> (resulting string=→"Total Channels":string)  [unwired: 2 in, 1 out]
            n45 = property on="Delete Type" class="Bool (strict)"("DisabledEnum"=w53) -> ()  [unwired: 2 in, 2 out]
            n46 = property on="# Parts" class="DigNum (strict)"("DisabledEnum"=w53) -> ()  [unwired: 2 in, 2 out]
            n47 = property on="# Signals" class="DigNum (strict)"("DisabledEnum"=w53) -> ()  [unwired: 2 in, 2 out]
            n48 = property on="Signals  Names" class="Arr (strict)"("DisabledEnum"=w53) -> ()  [unwired: 2 in, 2 out]
            n49 = property on="Signal" class="Clust (strict)"("DisabledEnum"=w53) -> ()  [unwired: 2 in, 2 out]
            n50 = property on="Rename" class="Bool (strict)"("DisabledEnum"=w53) -> ()  [unwired: 2 in, 2 out]
          }
          event "Rename": Value Change {
            # "Rename the Type"
            n51 = event-data() -> ()  [unwired: 1 in, 5 out]
            n52 = property on="Rename" class="Bool (strict)"("Value"=FALSE ("Rename")) -> ()  [unwired: 2 in, 2 out]
            n53 = Insert Into Array(array=w82, index=0, new element=string[] ["Rename", "Update Controls"]) -> (w83:string[])
          }
          event "# Parts": Value Change {
            # "Change the Number of Parts"
            n54 = event-data() -> ("NewVal"=w92:u16)  [unwired: 1 in]
            n55 = Unbundle By Name(w89) -> ("All Type Info"=w91:T10, "Type Index"=w94:i32)
            n56 = In Range and Coerce(upper limit=u16 8, x=w92, lower limit=u16 1) -> (coerced(x)=w95:u16, In Range?=w97:bool)
            n57 = Not(x=w97) -> (.not. x?=w96:bool)
            n58 = property on="Part Numbers" class="Arr (strict)"("Number of Rows"=w95, "VertScroll"=w96) -> ()  [unwired: 2 in, 2 out]
            n59 = Decrement(x=w94) -> (x-1=w86:i32)
            n60 = Index Array(array=w91, index=w86) -> (element=w93:T15)
            n61 = Bundle By Name(cluster=w93, "# Parts"=w92) -> (w90:T15)
            n62 = Replace Array Subset(array=w91, new element=w90, index=w86) -> (w87:T10)
            n63 = Bundle By Name(cluster=w89, "All Type Info"=w87) -> (w88:T12)
          }
          event "# Signals": Value Change {
            n64 = event-data() -> ("NewVal"=w100:u16)  [unwired: 1 in]
            n65 = In Range and Coerce(upper limit=u16 7, x=w100, lower limit=u16 1) -> (coerced(x)=w110:u16, In Range?=w112:bool)
            n66 = Unbundle By Name(w101) -> ("All Type Info"=w106:T10, "Type Index"=w108:i32)
            n67 = Not(x=w112) -> (.not. x?=w111:bool)
            n68 = property on="Signals  Names" class="Arr (strict)"("Number of Rows"=w110, "VertScroll"=w111) -> ()  [unwired: 2 in, 2 out]
            n69 = Decrement(x=w108) -> (x-1=w103:i32)
            n70 = Index Array(array=w106, index=w103) -> (element=w107:T15)
            n71 = Bundle By Name(cluster=w107, "# Signals"=w100) -> (w105:T15)
            n72 = Replace Array Subset(array=w106, new element=w105, index=w103) -> (w104:T10)
            n73 = Bundle By Name(cluster=w101, "All Type Info"=w104) -> (w102:T12)
          }
          event "Signals  Names": Value Change {
            # "Build Array of Buttons and New Array to Clear Buttons"
            n74 = event-data() -> ("NewVal"=w122:T1)  [unwired: 1 in]
            n75 = for {
              tunnel: w122 -> [w132] mode=indexing
              tunnel: [w131] -> w125 mode=indexing
              tunnel: [w129] -> w123 mode=indexing
              n76 = Unbundle By Name(w132) -> ("Signal Names"=w130:string, "Test Limits"=w131:bool)
              n77 = Bundle("Signal Names"=w130, "element"=FALSE) -> (w129:cluster{"Signal Names":string, "element":bool})  [unwired: 1 in]
            }
            n78 = property on="Signals  Names" class="Arr (strict)"("Value"=w123) -> ()  [unwired: 2 in, 2 out]
            n79 = Search 1D Array(1D array=w125, element=TRUE) -> (index of element=w115:i32)  [unwired: 1 in]
            n80 = case shown="Default" w115 {
              tunnel: [string[] [] string[] ["Load Test Limits", "Display Limits Tab"]] -> w121
              frame -1 {
              }
              frame Default {
              }
            }
            n81 = Bundle By Name(cluster=w117, "Test Limit Index"=w115) -> (w116:T12)
            n82 = Insert Into Array(array=w119, index=0, new element=w121) -> (w118:string[])
          }
          event "Signal Style": Value Change {
            n83 = event-data() -> ("NewVal"=w137:enum16{"Steady State", "Cyclic"}, "OldVal"=w133:enum16{"Steady State", "Cyclic"})  [unwired: 1 in]
            n84 = case shown="\"Cyclic\"" w137 {
              frame "Steady State" {
                n85 = property on="EU Low State Min" class="DigNum (strict)"("Visible"=FALSE, "Value"=0.0 ("EU High State Min")) -> ()  [unwired: 2 in, 2 out]
                n86 = property on="EU Low State Max" class="DigNum (strict)"("Visible"=FALSE, "Value"=0.0 ("EU High State Max")) -> ()  [unwired: 2 in, 2 out]
                n87 = property on="EU High State Max" class="DigNum (strict)"("Caption.Text"="EU Maximum" ("Label.Text")) -> ()  [unwired: 2 in, 2 out]
                n88 = property on="EU High State Min" class="DigNum (strict)"("Caption.Text"="EU Minimum" ("Label.Text")) -> ()  [unwired: 2 in, 2 out]
              }
              frame "Cyclic" {
                n89 = property on="EU Low State Min" class="DigNum (strict)"("Visible"=TRUE) -> ()  [unwired: 2 in, 2 out]
                n90 = property on="EU Low State Max" class="DigNum (strict)"("Visible"=TRUE) -> ()  [unwired: 2 in, 2 out]
                n91 = property on="EU High State Max" class="DigNum (strict)"("Caption.Text"="EU High State Max" ("Label.Text")) -> ()  [unwired: 2 in, 2 out]
                n92 = property on="EU High State Min" class="DigNum (strict)"("Caption.Text"="EU High State Min" ("Label.Text")) -> ()  [unwired: 2 in, 2 out]
              }
            }
            n93 = Bundle By Name(cluster=w136, "Signal Style Index"=w137, "Last Signal Style Index"=w133) -> (w135:T12)
          }
          event "Type": Value Change {
            n94 = event-data() -> ("NewVal"=w150:u16, "OldVal"=w148:u16)  [unwired: 1 in]
            n95 = Equal To 0?(x=w148) -> (x = 0?=w149:bool)
            n96 = case shown="False" w149 {
              tunnel: [string[] ["Switch Type", "Update Controls"] string[] ["Update Controls"]] -> w153
              frame False {
                # "Add Switch Type Case to Save Changes"
              }
              frame True {
                # "Do Not Save Changes"
              }
            }
            n97 = Bundle By Name(cluster=w152, "Type Index"=w150, "Last Type Index"=w148) -> (w151:T12)
            n98 = Insert Into Array(array=w155, index=0, new element=w153) -> (w156:string[])
          }
          event "Add New Type": Value Change {
            n99 = event-data() -> ()  [unwired: 1 in, 1 out]
            n100 = property on="Add New Type" class="Bool (strict)"("Value"=FALSE ("Add New Type")) -> ()  [unwired: 2 in, 2 out]
            n101 = Insert Into Array(array=w163, index=0, new element=string[] ["Add New Type", "Update Controls"]) -> (w164:string[])
          }
          event "Delete Type": Value Change {
            n102 = event-data() -> ()  [unwired: 1 in, 1 out]
            n103 = property on="Delete Type" class="Bool (strict)"("Value"=FALSE ("Delete Type")) -> ()  [unwired: 2 in, 2 out]
            n104 = Insert Into Array(array=w169, index=0, new element=string[] ["Delete Type", "Update Controls"]) -> (w170:string[])
          }
          event "OK": Value Change {
            n105 = event-data() -> ()  [unwired: 1 in, 1 out]
            n106 = property on="OK" class="Bool (strict)"("Value"=FALSE ("OK")) -> ()  [unwired: 2 in, 2 out]
            n107 = property on="Tab Control" class="TabCtl (strict)"() -> ("Value"=w173:enum32{"Main", "Limits"})  [unwired: 2 in, 2 out]
            n108 = case shown="\"Main\", Default" w173 {
              tunnel: [string[] ["Switch Type", "Check Config", "Build New Config", "Exit"] string[] ["Save Test Limits", "Display Main Tab"]] -> w176
              tunnel: w171 -> [w182 w184]
              tunnel: [w181 w184] -> w172
              tunnel: w171 -> [w180 _]
              frame "Main", Default {
                # "OK While Main Tab Open"
                # "Update Last Type Index and Call Switch type case.  This will save the current values of the controls on the screen"
                n109 = Unbundle By Name(w180) -> ("Type Index"=w179:i32)
                n110 = Bundle By Name(cluster=w182, "Last Type Index"=w179) -> (w181:T12)
              }
              frame "Limits" {
                # "OK While Limits Screen Open"
              }
            }
            n111 = Insert Into Array(array=w178, index=0, new element=w176) -> (w177:string[])
          }
          event "Cancel": Value Change {
            n112 = event-data() -> ()  [unwired: 1 in, 1 out]
            n113 = property on="Cancel" class="Bool (strict)"("Value"=FALSE ("Cancel")) -> ()  [unwired: 2 in, 2 out]
            n114 = property on="Tab Control" class="TabCtl (strict)"() -> ("Value"=w186:enum32{"Main", "Limits"})  [unwired: 2 in, 2 out]
            n115 = case shown="\"Main\", Default" w186 {
              tunnel: [string[] ["Exit"] string[] ["Display Main Tab"]] -> w189
              frame "Main", Default {
                # "Cancel While Main Tab Open"
              }
              frame "Limits" {
                # "Cancel While Limits Tab Open"
              }
            }
            n116 = Insert Into Array(array=w191, index=0, new element=w189) -> (w190:string[])
          }
          event Panel Close? {
            n117 = event-data() -> ()  [unwired: 1 in, 1 out]
            n118 = Insert Into Array(array=w199, index=0, new element=string[] ["Exit"]) -> (w198:string[])
            n119 = event-data("Discard?"=TRUE) -> ()  [unwired: 1 in, 1 out]
          }
        }
      }
      frame "Load Config" {
        # "Load the config file to the screen"
        n120 = Unbundle By Name(w206) -> ("Loaded Config"=w208:T2)
        n121 = Unbundle By Name(w208) -> ("All Type Info"=w202:T10, "Test Limits"=w207:T9[])
        n122 = call "Read Part Limits From Configuration.vi"("Test Limits"=w207, "All Part Info"=w202) -> ("Type Test Limits"=w204:cluster{T9[]}[])  [unwired: 9 in]
        n123 = call "Load Part Config Data.vi"("All Part Info"=w202) -> ("All Part Info Out"=w203:T16)  [unwired: 10 in]
        n124 = Array Size(array=w202) -> (size(s)=w201:i32)
        n125 = Bundle By Name(cluster=w206, "All Test Limits"=w204, "All Type Info"=w203, "Type Index"=w201) -> (w205:T12)
      }
      frame "Update Controls" {
        # "Update # Signals and Signals Names"
        # "Update # Parts and Part Numbers"
        # "Update Type Control"
        n126 = Unbundle By Name(w210) -> ("Type Index"=w217:i32, "All Type Info"=w223:T10)
        n127 = Unbundle By Name(w210) -> ("All Type Info"=w225:T10, "Type Index"=w224:i32)
        n128 = Decrement(x=w224) -> (x-1=w213:i32)
        n129 = for {
          tunnel: w223 -> [w235] mode=indexing
          tunnel: [w234] -> w216 mode=indexing
          n130 = Unbundle By Name(w235) -> ("Type Name"=w234:string)
        }
        n131 = Index Array(array=w225, index=w213) -> (element=w220:T15)
        n132 = Unbundle By Name(w220) -> ("# Signals"=w212:i32, "Type Signal Names"=w219:string[])
        n133 = Unbundle By Name(w220) -> ("# Parts"=w211:i32, "Part Info"=w222:T11[])
        n134 = Build Array (concatenate)("<NO SELECTION >", w216) -> (w214:string[])
        n135 = for {
          tunnel: w222 -> [w233] mode=indexing
          tunnel: [w230] -> w221 mode=indexing
          n136 = Unbundle(w233) -> ("Part Number"=w232:string, "Enabled?"=w231:bool)  [unwired: 1 out]
          n137 = Bundle("Part Number"=w232, "Enabled?"=w231) -> (w230:cluster{"Part Number":string, "Enabled?":bool})  [unwired: 1 in]
        }
        n138 = property on="Type" class="Ring (strict)"("Value"=w217, "Strings []"=w214) -> ()  [unwired: 2 in, 2 out]
        n139 = for {
          tunnel: w219 -> [w229] mode=indexing
          tunnel: [w227] -> w218 mode=indexing
          n140 = Bundle("Part Number"=w229, "Enabled?"=FALSE) -> (w227:cluster{"Part Number":string, "Enabled?":bool})  [unwired: 1 in]
        }
        n141 = property on="Signals  Names" class="Arr (strict)"("Number of Rows"=w212, "Value"=w218) -> ()  [unwired: 2 in, 2 out]
        n142 = property on="# Signals" class="DigNum (strict)"("Value"=w212) -> ()  [unwired: 2 in, 2 out]
        n143 = property on="Part Numbers" class="Arr (strict)"("Number of Rows"=w211, "Value"=w221) -> ()  [unwired: 2 in, 2 out]
        n144 = property on="# Parts" class="DigNum (strict)"("Value"=w211) -> ()  [unwired: 2 in, 2 out]
      }
      frame "Build New Config" {
        # "This VI takes the changes and Builds the channels with updates names"
        n145 = Unbundle By Name(w239) -> ("Loaded Config"=w236:T2, "Modified Config"=w242:T2, "All Type Info"=w241:T10, "All Test Limits"=w240:cluster{T9[]}[])
        n146 = call "Build Config File From Part Config.vi"("Loaded Config"=w236, "All Test Limits"=w240, "All Type Info"=w241, "Config In"=w242) -> ("Config Out"=w237:T2)  [unwired: 7 in]
        n147 = Bundle By Name(cluster=w239, "Modified Config"=w237) -> (w238:T12)
      }
      frame "Check Config" {
        # "Check for the following criteria:\n-Empty Signal Name\n-Too may signals defined\n-No Signals Defined\n-Empty Part Number"
        n148 = Unbundle By Name(w257) -> ("All Type Info"=w255:T10)
        n149 = for {
          tunnel: w255 -> [w277] mode=indexing
          shift-right: [w284] -> w247
          shift-left: 0 ("# Signals") -> [w285]
          tunnel: [w278] -> w253 mode=indexing
          tunnel: [w274] -> w245 mode=indexing
          n150 = Unbundle By Name(w277) -> ("Type Signal Names"=w280:string[], "# Signals"=w283:i32, "# Parts"=w282:i32)
          n151 = Unbundle By Name(w277) -> ("Part Info"=w276:T11[])
          n152 = for {
            tunnel: w276 -> [w288] mode=indexing
            tunnel: [w286] -> w275 mode=indexing
            n153 = Unbundle By Name(w288) -> ("Part Number"=w287:string)
            n154 = Empty String/Path?(string/path=w287) -> (empty?=w286:bool)
          }
          n155 = Multiply(x=w283, y=w282) -> (x*y=w281:i32)
          n156 = for {
            tunnel: w280 -> [w290] mode=indexing
            tunnel: [w289] -> w279 mode=indexing
            n157 = Empty String/Path?(string/path=w290) -> (empty?=w289:bool)
          }
          n158 = Add(x=w281, y=w285) -> (x+y=w284:i32)
          n159 = Or Array Elements(Boolean array=w279) -> (logical OR=w278:bool)
          n160 = Or Array Elements(Boolean array=w275) -> (logical OR=w274:bool)
        }
        n161 = Or Array Elements(Boolean array=w253) -> (logical OR=w249:bool)
        n162 = Or Array Elements(Boolean array=w245) -> (logical OR=w244:bool)
        n163 = Greater?(x=w247, y=32) -> (0:w248:bool)
        n164 = Less Or Equal To 0?(x=w247) -> (x <= 0?=w246:bool)
        n165 = Compound Arithmetic op=OR(w249, w248, w246, w244) -> (w251:bool)
        n166 = case shown="True" w251 {
          tunnel: w252 -> [w258 _]
          tunnel: [w258 string[] []] -> w250
          tunnel: w249 -> [_ w268]
          tunnel: w248 -> [_ w267]
          tunnel: w246 -> [_ w261]
          tunnel: w244 -> [_ w259]
          frame False {
          }
          frame True {
            n167 = case shown="True" w267 {
              tunnel: [_ "- Too many channels defined\n"] -> w263
              frame False {
              }
              frame True {
              }
            }
            n168 = case shown="True" w261 {
              tunnel: [_ "- No channels defined\n"] -> w260
              frame False {
              }
              frame True {
              }
            }
            n169 = case shown="True" w259 {
              tunnel: [_ "- A part does not have a name.\n"] -> _
              frame False {
              }
              frame True {
              }
            }
            n170 = case shown="True" w268 {
              tunnel: [_ "- A signal does not have a name.\n"] -> w264
              frame False {
              }
              frame True {
              }
            }
            n171 = Concatenate Strings(w264, w263, w260) -> (w262:string)
            n172 = Format Into String(format string="Configuration error detected:\n\n%s", w262) -> (resulting string=w265:string)  [unwired: 2 in, 1 out]
            n173 = One Button Dialog(message=w265) -> ()  [unwired: 1 in, 1 out]
          }
        }
      }
      frame "Switch Type" {
        n174 = Unbundle By Name(w297) -> ("All Type Info"=w300:T10, "Last Type Index"=w305:i32)
        n175 = Decrement(x=w305) -> (x-1=w299:i32)
        n176 = Index Array(array=w300, index=w299) -> (element=w302:T15)
        n177 = Unbundle By Name(w302) -> ("Part Info"=w304:T11[])
        n178 = for {
          tunnel: w304 -> [w312] mode=indexing
          tunnel: w303 -> [w313] mode=indexing
          tunnel: [w310] -> w301 mode=indexing
          n179 = Unbundle(w313) -> ("Part Number"=w311:string, "Acquire"=w309:bool)
          n180 = Bundle By Name(cluster=w312, "Part Number"=w311, "Enabled?"=w309) -> (w310:T11)
        }
        n181 = for {
          tunnel: w294 -> [w308] mode=indexing
          tunnel: [w307] -> w293 mode=indexing
          n182 = Unbundle(w308) -> ("Signal Names"=w307:string)  [unwired: 1 out]
        }
        n183 = Bundle By Name(cluster=w302, "Part Info"=w301, "Type Signal Names"=w293, "# Parts"=w292, "# Signals"=w291) -> (w298:T15)
        n184 = Replace Array Subset(array=w300, new element=w298, index=w299) -> (w295:T10)
        n185 = Bundle By Name(cluster=w297, "All Type Info"=w295) -> (w296:T12)
      }
      frame "Add New Type" {
        n186 = Unbundle By Name(w319) -> ("All Test Limits"=w318:cluster{T9[]}[])
        n187 = Unbundle By Name(w319) -> ("Type Index"=w316:i32, "All Type Info"=w323:T10)
        n188 = call "Type Name Dialog.vi"("Type Name:"="New Type" ("Type Name In")) -> ("Type Name Out"=w322:string, "Cancelled?"=w314:bool)  [unwired: 13 in]
        n189 = case shown="False" w314 {
          tunnel: w323 -> [w340 w342]
          tunnel: w322 -> [w338 _]
          tunnel: [w335 w342] -> w320
          tunnel: w318 -> [w333 w341]
          tunnel: [w331 w341] -> w317
          tunnel: w316 -> [w330 w343]
          tunnel: [w329 w343] -> w315
          frame False {
            w336 = 1 ("# Signals")
            # "Add New Part"
            n190 = Bundle By Name(cluster=T14 {"Type Name"="", "Type Signal Names"=[], "# Signals"=0, "# Parts"=0, "Type Info"=[]} ("new element/subarray"), "Type Name"=w338, "Type Signal Names"=string[] ["Signal 1", "Signal 2", "Signal 3", "Signal 4", "Signal 5", "Signal 6", "Signal 7", "Signal 8", "Signal 9", "Signal 10", "Signal 11", "Signal 12", "Signal 13", "Signal 14", "Signal 15", "Signal 16", "Signal 17", "Signal 18", "Signal 19", "Signal 20", "Signal 21", "Signal 22", "Signal 23", "Signal 24", "Signal 25", "Signal 26", "Signal 27", "Signal 28", "Signal 29", "Signal 30", "Signal 31", "Signal 32"] ("Array"), "# Signals"=w336, "# Parts"=w336, "Type Info"=T11[] [{"Part Number"="Part 1", "Channel Indexes"=[], "Enabled?"=FALSE}, {"Part Number"="Part 2", "Channel Indexes"=[], "Enabled?"=FALSE}, {"Part Number"="Part 3", "Channel Indexes"=[], "Enabled?"=FALSE}, {"Part Number"="Part 4", "Channel Indexes"=[], "Enabled?"=FALSE}, {"Part Number"="Part 5", "Channel Indexes"=[], "Enabled?"=FALSE}, {"Part Number"="Part 6", "Channel Indexes"=[], "Enabled?"=FALSE}, {"Part Number"="Part 7", "Channel Indexes"=[], "Enabled?"=FALSE}, {"Part Number"="Part 8", "Channel Indexes"=[], "Enabled?"=FALSE}, {"Part Number"="Part 9", "Channel Indexes"=[], "Enabled?"=FALSE}, {"Part Number"="Part 10", "Channel Indexes"=[], "Enabled?"=FALSE}, {"Part Number"="Part 11", "Channel Indexes"=[], "Enabled?"=FALSE}, {"Part Number"="Part 12", "Channel Indexes"=[], "Enabled?"=FALSE}, {"Part Number"="Part 13", "Channel Indexes"=[], "Enabled?"=FALSE}, {"Part Number"="Part 14", "Channel Indexes"=[], "Enabled?"=FALSE}, {"Part Number"="Part 15", "Channel Indexes"=[], "Enabled?"=FALSE}, {"Part Number"="Part 16", "Channel Indexes"=[], "Enabled?"=FALSE}, {"Part Number"="Part 17", "Channel Indexes"=[], "Enabled?"=FALSE}, {"Part Number"="Part 18", "Channel Indexes"=[], "Enabled?"=FALSE}, {"Part Number"="Part 19", "Channel Indexes"=[], "Enabled?"=FALSE}, {"Part Number"="Part 20", "Channel Indexes"=[], "Enabled?"=FALSE}, {"Part Number"="Part 21", "Channel Indexes"=[], "Enabled?"=FALSE}, {"Part Number"="Part 22", "Channel Indexes"=[], "Enabled?"=FALSE}, {"Part Number"="Part 23", "Channel Indexes"=[], "Enabled?"=FALSE}, {"Part Number"="Part 24", "Channel Indexes"=[], "Enabled?"=FALSE}, {"Part Number"="Part 25", "Channel Indexes"=[], "Enabled?"=FALSE}, {"Part Number"="Part 26", "Channel Indexes"=[], "Enabled?"=FALSE}, {"Part Number"="Part 27", "Channel Indexes"=[], "Enabled?"=FALSE}, {"Part Number"="Part 28", "Channel Indexes"=[], "Enabled?"=FALSE}, {"Part Number"="Part 29", "Channel Indexes"=[], "Enabled?"=FALSE}, {"Part Number"="Part 30", "Channel Indexes"=[], "Enabled?"=FALSE}, {"Part Number"="Part 31", "Channel Indexes"=[], "Enabled?"=FALSE}, {"Part Number"="Part 32", "Channel Indexes"=[], "Enabled?"=FALSE}] ("Array")) -> (w337:T14)
            n191 = Array Size(array=w340) -> (size(s)=w328:i32)
            n192 = Array Size(array=w333) -> (size(s)=w334:i32)
            n193 = Increment(x=w330) -> (x+1=w329:i32)
            n194 = Insert Into Array(array=w340, index=w328, new element=w337) -> (w335:T10)
            n195 = Insert Into Array(array=w333, index=w334, new element=cluster{T9[]} {[{"Channel Acquired?"=FALSE, "RMS?"=FALSE, "Pk-Pk"=FALSE, "Frequency"=FALSE, "EU High Limit 1"=0.0, "EU Low Limit 1"=0.0, "EU High Limit 2"=0.0, "EU Low Limit 2"=0.0, "RMS High Limit"=0.0, "RMS Low Limit"=0.0, "Pk-Pk High Limit "=0.0, "Pk-Pk Low Limit"=0.0, "Frequency High Limit"=0.0, "Frequency Low Limit"=0.0}, {"Channel Acquired?"=FALSE, "RMS?"=FALSE, "Pk-Pk"=FALSE, "Frequency"=FALSE, "EU High Limit 1"=0.0, "EU Low Limit 1"=0.0, "EU High Limit 2"=0.0, "EU Low Limit 2"=0.0, "RMS High Limit"=0.0, "RMS Low Limit"=0.0, "Pk-Pk High Limit "=0.0, "Pk-Pk Low Limit"=0.0, "Frequency High Limit"=0.0, "Frequency Low Limit"=0.0}, {"Channel Acquired?"=FALSE, "RMS?"=FALSE, "Pk-Pk"=FALSE, "Frequency"=FALSE, "EU High Limit 1"=0.0, "EU Low Limit 1"=0.0, "EU High Limit 2"=0.0, "EU Low Limit 2"=0.0, "RMS High Limit"=0.0, "RMS Low Limit"=0.0, "Pk-Pk High Limit "=0.0, "Pk-Pk Low Limit"=0.0, "Frequency High Limit"=0.0, "Frequency Low Limit"=0.0}, {"Channel Acquired?"=FALSE, "RMS?"=FALSE, "Pk-Pk"=FALSE, "Frequency"=FALSE, "EU High Limit 1"=0.0, "EU Low Limit 1"=0.0, "EU High Limit 2"=0.0, "EU Low Limit 2"=0.0, "RMS High Limit"=0.0, "RMS Low Limit"=0.0, "Pk-Pk High Limit "=0.0, "Pk-Pk Low Limit"=0.0, "Frequency High Limit"=0.0, "Frequency Low Limit"=0.0}, {"Channel Acquired?"=FALSE, "RMS?"=FALSE, "Pk-Pk"=FALSE, "Frequency"=FALSE, "EU High Limit 1"=0.0, "EU Low Limit 1"=0.0, "EU High Limit 2"=0.0, "EU Low Limit 2"=0.0, "RMS High Limit"=0.0, "RMS Low Limit"=0.0, "Pk-Pk High Limit "=0.0, "Pk-Pk Low Limit"=0.0, "Frequency High Limit"=0.0, "Frequency Low Limit"=0.0}, {"Channel Acquired?"=FALSE, "RMS?"=FALSE, "Pk-Pk"=FALSE, "Frequency"=FALSE, "EU High Limit 1"=0.0, "EU Low Limit 1"=0.0, "EU High Limit 2"=0.0, "EU Low Limit 2"=0.0, "RMS High Limit"=0.0, "RMS Low Limit"=0.0, "Pk-Pk High Limit "=0.0, "Pk-Pk Low Limit"=0.0, "Frequency High Limit"=0.0, "Frequency Low Limit"=0.0}, {"Channel Acquired?"=FALSE, "RMS?"=FALSE, "Pk-Pk"=FALSE, "Frequency"=FALSE, "EU High Limit 1"=0.0, "EU Low Limit 1"=0.0, "EU High Limit 2"=0.0, "EU Low Limit 2"=0.0, "RMS High Limit"=0.0, "RMS Low Limit"=0.0, "Pk-Pk High Limit "=0.0, "Pk-Pk Low Limit"=0.0, "Frequency High Limit"=0.0, "Frequency Low Limit"=0.0}, {"Channel Acquired?"=FALSE, "RMS?"=FALSE, "Pk-Pk"=FALSE, "Frequency"=FALSE, "EU High Limit 1"=0.0, "EU Low Limit 1"=0.0, "EU High Limit 2"=0.0, "EU Low Limit 2"=0.0, "RMS High Limit"=0.0, "RMS Low Limit"=0.0, "Pk-Pk High Limit "=0.0, "Pk-Pk Low Limit"=0.0, "Frequency High Limit"=0.0, "Frequency Low Limit"=0.0}, {"Channel Acquired?"=FALSE, "RMS?"=FALSE, "Pk-Pk"=FALSE, "Frequency"=FALSE, "EU High Limit 1"=0.0, "EU Low Limit 1"=0.0, "EU High Limit 2"=0.0, "EU Low Limit 2"=0.0, "RMS High Limit"=0.0, "RMS Low Limit"=0.0, "Pk-Pk High Limit "=0.0, "Pk-Pk Low Limit"=0.0, "Frequency High Limit"=0.0, "Frequency Low Limit"=0.0}, {"Channel Acquired?"=FALSE, "RMS?"=FALSE, "Pk-Pk"=FALSE, "Frequency"=FALSE, "EU High Limit 1"=0.0, "EU Low Limit 1"=0.0, "EU High Limit 2"=0.0, "EU Low Limit 2"=0.0, "RMS High Limit"=0.0, "RMS Low Limit"=0.0, "Pk-Pk High Limit "=0.0, "Pk-Pk Low Limit"=0.0, "Frequency High Limit"=0.0, "Frequency Low Limit"=0.0}, {"Channel Acquired?"=FALSE, "RMS?"=FALSE, "Pk-Pk"=FALSE, "Frequency"=FALSE, "EU High Limit 1"=0.0, "EU Low Limit 1"=0.0, "EU High Limit 2"=0.0, "EU Low Limit 2"=0.0, "RMS High Limit"=0.0, "RMS Low Limit"=0.0, "Pk-Pk High Limit "=0.0, "Pk-Pk Low Limit"=0.0, "Frequency High Limit"=0.0, "Frequency Low Limit"=0.0}, {"Channel Acquired?"=FALSE, "RMS?"=FALSE, "Pk-Pk"=FALSE, "Frequency"=FALSE, "EU High Limit 1"=0.0, "EU Low Limit 1"=0.0, "EU High Limit 2"=0.0, "EU Low Limit 2"=0.0, "RMS High Limit"=0.0, "RMS Low Limit"=0.0, "Pk-Pk High Limit "=0.0, "Pk-Pk Low Limit"=0.0, "Frequency High Limit"=0.0, "Frequency Low Limit"=0.0}, {"Channel Acquired?"=FALSE, "RMS?"=FALSE, "Pk-Pk"=FALSE, "Frequency"=FALSE, "EU High Limit 1"=0.0, "EU Low Limit 1"=0.0, "EU High Limit 2"=0.0, "EU Low Limit 2"=0.0, "RMS High Limit"=0.0, "RMS Low Limit"=0.0, "Pk-Pk High Limit "=0.0, "Pk-Pk Low Limit"=0.0, "Frequency High Limit"=0.0, "Frequency Low Limit"=0.0}, {"Channel Acquired?"=FALSE, "RMS?"=FALSE, "Pk-Pk"=FALSE, "Frequency"=FALSE, "EU High Limit 1"=0.0, "EU Low Limit 1"=0.0, "EU High Limit 2"=0.0, "EU Low Limit 2"=0.0, "RMS High Limit"=0.0, "RMS Low Limit"=0.0, "Pk-Pk High Limit "=0.0, "Pk-Pk Low Limit"=0.0, "Frequency High Limit"=0.0, "Frequency Low Limit"=0.0}, {"Channel Acquired?"=FALSE, "RMS?"=FALSE, "Pk-Pk"=FALSE, "Frequency"=FALSE, "EU High Limit 1"=0.0, "EU Low Limit 1"=0.0, "EU High Limit 2"=0.0, "EU Low Limit 2"=0.0, "RMS High Limit"=0.0, "RMS Low Limit"=0.0, "Pk-Pk High Limit "=0.0, "Pk-Pk Low Limit"=0.0, "Frequency High Limit"=0.0, "Frequency Low Limit"=0.0}, {"Channel Acquired?"=FALSE, "RMS?"=FALSE, "Pk-Pk"=FALSE, "Frequency"=FALSE, "EU High Limit 1"=0.0, "EU Low Limit 1"=0.0, "EU High Limit 2"=0.0, "EU Low Limit 2"=0.0, "RMS High Limit"=0.0, "RMS Low Limit"=0.0, "Pk-Pk High Limit "=0.0, "Pk-Pk Low Limit"=0.0, "Frequency High Limit"=0.0, "Frequency Low Limit"=0.0}, {"Channel Acquired?"=FALSE, "RMS?"=FALSE, "Pk-Pk"=FALSE, "Frequency"=FALSE, "EU High Limit 1"=0.0, "EU Low Limit 1"=0.0, "EU High Limit 2"=0.0, "EU Low Limit 2"=0.0, "RMS High Limit"=0.0, "RMS Low Limit"=0.0, "Pk-Pk High Limit "=0.0, "Pk-Pk Low Limit"=0.0, "Frequency High Limit"=0.0, "Frequency Low Limit"=0.0}, {"Channel Acquired?"=FALSE, "RMS?"=FALSE, "Pk-Pk"=FALSE, "Frequency"=FALSE, "EU High Limit 1"=0.0, "EU Low Limit 1"=0.0, "EU High Limit 2"=0.0, "EU Low Limit 2"=0.0, "RMS High Limit"=0.0, "RMS Low Limit"=0.0, "Pk-Pk High Limit "=0.0, "Pk-Pk Low Limit"=0.0, "Frequency High Limit"=0.0, "Frequency Low Limit"=0.0}, {"Channel Acquired?"=FALSE, "RMS?"=FALSE, "Pk-Pk"=FALSE, "Frequency"=FALSE, "EU High Limit 1"=0.0, "EU Low Limit 1"=0.0, "EU High Limit 2"=0.0, "EU Low Limit 2"=0.0, "RMS High Limit"=0.0, "RMS Low Limit"=0.0, "Pk-Pk High Limit "=0.0, "Pk-Pk Low Limit"=0.0, "Frequency High Limit"=0.0, "Frequency Low Limit"=0.0}, {"Channel Acquired?"=FALSE, "RMS?"=FALSE, "Pk-Pk"=FALSE, "Frequency"=FALSE, "EU High Limit 1"=0.0, "EU Low Limit 1"=0.0, "EU High Limit 2"=0.0, "EU Low Limit 2"=0.0, "RMS High Limit"=0.0, "RMS Low Limit"=0.0, "Pk-Pk High Limit "=0.0, "Pk-Pk Low Limit"=0.0, "Frequency High Limit"=0.0, "Frequency Low Limit"=0.0}, {"Channel Acquired?"=FALSE, "RMS?"=FALSE, "Pk-Pk"=FALSE, "Frequency"=FALSE, "EU High Limit 1"=0.0, "EU Low Limit 1"=0.0, "EU High Limit 2"=0.0, "EU Low Limit 2"=0.0, "RMS High Limit"=0.0, "RMS Low Limit"=0.0, "Pk-Pk High Limit "=0.0, "Pk-Pk Low Limit"=0.0, "Frequency High Limit"=0.0, "Frequency Low Limit"=0.0}, {"Channel Acquired?"=FALSE, "RMS?"=FALSE, "Pk-Pk"=FALSE, "Frequency"=FALSE, "EU High Limit 1"=0.0, "EU Low Limit 1"=0.0, "EU High Limit 2"=0.0, "EU Low Limit 2"=0.0, "RMS High Limit"=0.0, "RMS Low Limit"=0.0, "Pk-Pk High Limit "=0.0, "Pk-Pk Low Limit"=0.0, "Frequency High Limit"=0.0, "Frequency Low Limit"=0.0}, {"Channel Acquired?"=FALSE, "RMS?"=FALSE, "Pk-Pk"=FALSE, "Frequency"=FALSE, "EU High Limit 1"=0.0, "EU Low Limit 1"=0.0, "EU High Limit 2"=0.0, "EU Low Limit 2"=0.0, "RMS High Limit"=0.0, "RMS Low Limit"=0.0, "Pk-Pk High Limit "=0.0, "Pk-Pk Low Limit"=0.0, "Frequency High Limit"=0.0, "Frequency Low Limit"=0.0}, {"Channel Acquired?"=FALSE, "RMS?"=FALSE, "Pk-Pk"=FALSE, "Frequency"=FALSE, "EU High Limit 1"=0.0, "EU Low Limit 1"=0.0, "EU High Limit 2"=0.0, "EU Low Limit 2"=0.0, "RMS High Limit"=0.0, "RMS Low Limit"=0.0, "Pk-Pk High Limit "=0.0, "Pk-Pk Low Limit"=0.0, "Frequency High Limit"=0.0, "Frequency Low Limit"=0.0}, {"Channel Acquired?"=FALSE, "RMS?"=FALSE, "Pk-Pk"=FALSE, "Frequency"=FALSE, "EU High Limit 1"=0.0, "EU Low Limit 1"=0.0, "EU High Limit 2"=0.0, "EU Low Limit 2"=0.0, "RMS High Limit"=0.0, "RMS Low Limit"=0.0, "Pk-Pk High Limit "=0.0, "Pk-Pk Low Limit"=0.0, "Frequency High Limit"=0.0, "Frequency Low Limit"=0.0}, {"Channel Acquired?"=FALSE, "RMS?"=FALSE, "Pk-Pk"=FALSE, "Frequency"=FALSE, "EU High Limit 1"=0.0, "EU Low Limit 1"=0.0, "EU High Limit 2"=0.0, "EU Low Limit 2"=0.0, "RMS High Limit"=0.0, "RMS Low Limit"=0.0, "Pk-Pk High Limit "=0.0, "Pk-Pk Low Limit"=0.0, "Frequency High Limit"=0.0, "Frequency Low Limit"=0.0}, {"Channel Acquired?"=FALSE, "RMS?"=FALSE, "Pk-Pk"=FALSE, "Frequency"=FALSE, "EU High Limit 1"=0.0, "EU Low Limit 1"=0.0, "EU High Limit 2"=0.0, "EU Low Limit 2"=0.0, "RMS High Limit"=0.0, "RMS Low Limit"=0.0, "Pk-Pk High Limit "=0.0, "Pk-Pk Low Limit"=0.0, "Frequency High Limit"=0.0, "Frequency Low Limit"=0.0}, {"Channel Acquired?"=FALSE, "RMS?"=FALSE, "Pk-Pk"=FALSE, "Frequency"=FALSE, "EU High Limit 1"=0.0, "EU Low Limit 1"=0.0, "EU High Limit 2"=0.0, "EU Low Limit 2"=0.0, "RMS High Limit"=0.0, "RMS Low Limit"=0.0, "Pk-Pk High Limit "=0.0, "Pk-Pk Low Limit"=0.0, "Frequency High Limit"=0.0, "Frequency Low Limit"=0.0}, {"Channel Acquired?"=FALSE, "RMS?"=FALSE, "Pk-Pk"=FALSE, "Frequency"=FALSE, "EU High Limit 1"=0.0, "EU Low Limit 1"=0.0, "EU High Limit 2"=0.0, "EU Low Limit 2"=0.0, "RMS High Limit"=0.0, "RMS Low Limit"=0.0, "Pk-Pk High Limit "=0.0, "Pk-Pk Low Limit"=0.0, "Frequency High Limit"=0.0, "Frequency Low Limit"=0.0}, {"Channel Acquired?"=FALSE, "RMS?"=FALSE, "Pk-Pk"=FALSE, "Frequency"=FALSE, "EU High Limit 1"=0.0, "EU Low Limit 1"=0.0, "EU High Limit 2"=0.0, "EU Low Limit 2"=0.0, "RMS High Limit"=0.0, "RMS Low Limit"=0.0, "Pk-Pk High Limit "=0.0, "Pk-Pk Low Limit"=0.0, "Frequency High Limit"=0.0, "Frequency Low Limit"=0.0}, {"Channel Acquired?"=FALSE, "RMS?"=FALSE, "Pk-Pk"=FALSE, "Frequency"=FALSE, "EU High Limit 1"=0.0, "EU Low Limit 1"=0.0, "EU High Limit 2"=0.0, "EU Low Limit 2"=0.0, "RMS High Limit"=0.0, "RMS Low Limit"=0.0, "Pk-Pk High Limit "=0.0, "Pk-Pk Low Limit"=0.0, "Frequency High Limit"=0.0, "Frequency Low Limit"=0.0}, {"Channel Acquired?"=FALSE, "RMS?"=FALSE, "Pk-Pk"=FALSE, "Frequency"=FALSE, "EU High Limit 1"=0.0, "EU Low Limit 1"=0.0, "EU High Limit 2"=0.0, "EU Low Limit 2"=0.0, "RMS High Limit"=0.0, "RMS Low Limit"=0.0, "Pk-Pk High Limit "=0.0, "Pk-Pk Low Limit"=0.0, "Frequency High Limit"=0.0, "Frequency Low Limit"=0.0}]} ("new element/subarray")) -> (w331:cluster{T9[]}[])
          }
          frame True {
            # "Cancelled"
          }
        }
        n196 = Bundle By Name(cluster=w319, "Type Index"=w315, "All Type Info"=w320, "All Test Limits"=w317) -> (w321:T12)
      }
      frame "Delete Type" {
        n197 = Unbundle By Name(w350) -> ("All Test Limits"=w348:cluster{T9[]}[])
        n198 = Unbundle By Name(w350) -> ("Type Index"=w345:i32, "All Type Info"=w349:T10)
        n199 = Decrement(x=w345) -> (x-1=w344:i32)
        n200 = Delete From Array(array=w349, index=w344) -> (array with subset deleted=w347:T10)  [unwired: 1 in, 1 out]
        n201 = Delete From Array(array=w348, index=w344) -> (array with subset deleted=w346:cluster{T9[]}[])  [unwired: 1 in, 1 out]
        n202 = Bundle By Name(cluster=w350, "Type Index"=w344, "All Type Info"=w347, "All Test Limits"=w346) -> (w351:T12)
      }
      frame "Rename" {
        n203 = Unbundle By Name(w357) -> ("All Type Info"=w355:T10, "Type Index"=w361:i32)
        n204 = Decrement(x=w361) -> (x-1=w354:i32)
        n205 = Index Array(array=w355, index=w354) -> (element=w353:T15)
        n206 = Unbundle By Name(w353) -> ("Type Name"=w360:string)
        n207 = call "Type Name Dialog.vi"("Type Name:"=w360) -> ("Type Name Out"=w358:string, "Cancelled?"=w359:bool)  [unwired: 13 in]
        n208 = case shown="True" w359 {
          tunnel: w358 -> [w365 _]
          tunnel: w357 -> [w369 w371]
          tunnel: [w370 w371] -> w356
          tunnel: w355 -> [w368 _]
          tunnel: w354 -> [w367 _]
          tunnel: w353 -> [w366 _]
          frame False {
            n209 = Bundle By Name(cluster=w366, "Type Name"=w365) -> (w364:T15)
            n210 = Replace Array Subset(array=w368, new element=w364, index=w367) -> (w363:T10)
            n211 = Bundle By Name(cluster=w369, "All Type Info"=w363) -> (w370:T12)
          }
          frame True {
          }
        }
      }
      frame "Load Test Limits" {
        n212 = Unbundle By Name(w401) -> ("All Test Limits"=w399:cluster{T9[]}[], "Type Index"=w400:i32, "Test Limit Index"=w384:i32)
        n213 = for {
          tunnel: w386 -> [w410] mode=indexing
          tunnel: [w409] -> w383 mode=indexing
          n214 = Unbundle By Name(w410) -> ("Signal Names"=w409:string)
        }
        n215 = Decrement(x=w400) -> (x-1=w398:i32)
        n216 = Index Array(array=w399, index=w398) -> (element=w397:cluster{T9[]})
        n217 = Unbundle(w397) -> (w385:T9[])
        n218 = Index Array(array=w385, index=w384) -> (element=w387:T9)
        n219 = Index Array(array=w383, index=w384) -> (element=w380:string)
        n220 = Empty String/Path?(string/path=w380) -> (empty?=w382:bool)
        n221 = Unbundle By Name(w387) -> ("RMS?"=w395:bool, "Pk-Pk"=w394:bool, "Frequency"=w393:bool, "EU High Limit 2"=w377:dbl, "EU Low Limit 2"=w376:dbl, "EU High Limit 1"=w375:dbl, "EU Low Limit 1"=w374:dbl, "RMS High Limit"=w392:dbl, "RMS Low Limit"=w391:dbl, "Pk-Pk High Limit"=w390:dbl, "Pk-Pk Low Limit"=w389:dbl, "Frequency High Limit"=w388:dbl, "Frequency Low Limit"=w396:dbl)
        n222 = Select(t="No Signal Name", s=w382, f=w380) -> (s? t:f=→"Current Limit Selection:":string)
        n223 = Equal?(x=w375, y=w374) -> (x = y?=w378:bool)
        n224 = case shown="False" w378 {
          tunnel: [w405 w407] -> w373
          tunnel: [w405 w407] -> w372
          frame False {
            w405 = TRUE
            n225 = property on="EU High State Max" class="DigNum (strict)"("Caption.Text"="EU High State Max") -> ()  [unwired: 2 in, 2 out]
            n226 = property on="EU High State Min" class="DigNum (strict)"("Caption.Text"="EU High State Min") -> ()  [unwired: 2 in, 2 out]
            n227 = property on="Signal Style" class="Enum (strict)"("Value"=enum16{"Steady State", "Cyclic"}."Cyclic" ("Signal Style")) -> ()  [unwired: 2 in, 2 out]
          }
          frame True {
            w407 = FALSE
            n228 = property on="Signal Style" class="Enum (strict)"("Value"=enum16{"Steady State", "Cyclic"}."Steady State" ("Signal Style")) -> ()  [unwired: 2 in, 2 out]
          }
        }
        n229 = property on="Enable Limits" class="Bool (strict)"("Value"=w395) -> ()  [unwired: 2 in, 2 out]
        n230 = property on="Enable Limits" class="Bool (strict)"("Value"=w394) -> ()  [unwired: 2 in, 2 out]
        n231 = property on="Enable Limits" class="Bool (strict)"("Value"=w393) -> ()  [unwired: 2 in, 2 out]
        n232 = property on="EU High State Max" class="DigNum (strict)"("Value"=w377) -> ()  [unwired: 2 in, 2 out]
        n233 = property on="EU High State Min" class="DigNum (strict)"("Value"=w376) -> ()  [unwired: 2 in, 2 out]
        n234 = property on="EU Low State Max" class="DigNum (strict)"("Value"=w375) -> ()  [unwired: 2 in, 2 out]
        n235 = property on="EU Low State Min" class="DigNum (strict)"("Value"=w374) -> ()  [unwired: 2 in, 2 out]
        n236 = property on="RMS Maximum" class="DigNum (strict)"("Value"=w392) -> ()  [unwired: 2 in, 2 out]
        n237 = property on="RMS Minimum" class="DigNum (strict)"("Value"=w391) -> ()  [unwired: 2 in, 2 out]
        n238 = property on="Pk-Pk Maximum" class="DigNum (strict)"("Value"=w390) -> ()  [unwired: 2 in, 2 out]
        n239 = property on="Pk-Pk Minimum" class="DigNum (strict)"("Value"=w389) -> ()  [unwired: 2 in, 2 out]
        n240 = property on="Freq Maximum" class="DigNum (strict)"("Value"=w388) -> ()  [unwired: 2 in, 2 out]
        n241 = property on="Freq Minimum" class="DigNum (strict)"("Value"=w396) -> ()  [unwired: 2 in, 2 out]
        n242 = property on="EU Low State Min" class="DigNum (strict)"("Visible"=w373) -> ()  [unwired: 2 in, 2 out]
        n243 = property on="EU Low State Max" class="DigNum (strict)"("Visible"=w372) -> ()  [unwired: 2 in, 2 out]
      }
      frame "Save Test Limits" {
        n244 = Unbundle By Name(w413) -> ("All Test Limits"=w415:cluster{T9[]}[], "Type Index"=w436:i32, "Test Limit Index"=w418:i32)
        n245 = Decrement(x=w436) -> (x-1=w414:i32)
        n246 = Index Array(array=w415, index=w414) -> (element=w435:cluster{T9[]})
        n247 = Unbundle(w435) -> (w419:T9[])
        n248 = Index Array(array=w419, index=w418) -> (element=w434:T9)
        n249 = Bundle By Name(cluster=w434, "RMS?"="Enable Limits", "Pk-Pk"="Enable Limits", "Frequency"="Enable Limits", "EU High Limit 2"="EU High State Max", "EU Low Limit 2"="EU High State Min", "EU High Limit 1"="EU Low State Max", "EU Low Limit 1"="EU Low State Min", "RMS High Limit"="RMS Maximum", "RMS Low Limit"="RMS Minimum", "Pk-Pk High Limit"="Pk-Pk Maximum", "Pk-Pk Low Limit"="Pk-Pk Minimum", "Frequency High Limit"="Freq Maximum", "Frequency Low Limit"="Freq Minimum") -> (w420:T9)
        n250 = Replace Array Subset(array=w419, new element=w420, index=w418) -> (w417:T9[])
        n251 = Bundle(w417) -> (w416:cluster{T9[]})  [unwired: 1 in]
        n252 = Replace Array Subset(array=w415, new element=w416, index=w414) -> (w411:cluster{T9[]}[])
        n253 = Bundle By Name(cluster=w413, "All Test Limits"=w411) -> (w412:T12)
      }
      frame "Display Limits Tab" {
        w438 = T13."Disabled and Grayed Out" ("Disabled")
        n254 = property on="Type" class="Ring (strict)"("DisabledEnum"=w438) -> ()  [unwired: 2 in, 2 out]
        n255 = property on="Add New Type" class="Bool (strict)"("DisabledEnum"=w438) -> ()  [unwired: 2 in, 2 out]
        n256 = property on="Tab Control" class="TabCtl (strict)"("Value"=enum32{"Main", "Limits"}."Limits" ("Tab Control")) -> ()  [unwired: 2 in, 2 out]
      }
      frame "Display Main Tab" {
        n257 = property on="Type" class="Ring (strict)"("DisabledEnum"=T13."Enabled" ("Disabled")) -> ()  [unwired: 2 in, 2 out]
        n258 = property on="Add New Type" class="Bool (strict)"("DisabledEnum"=T13."Enabled" ("Disabled")) -> ()  [unwired: 2 in, 2 out]
        n259 = property on="Tab Control" class="TabCtl (strict)"("Value"=enum32{"Main", "Limits"}."Main" ("Tab Control")) -> ()  [unwired: 2 in, 2 out]
      }
      frame "Exit" {
      }
    }
  }
  n260 = flat-sequence {
    tunnel: w2 -> [_]
    tunnel: w1 -> [w453]
    frame #0 {
      # "Exit"
      n261 = Unbundle By Name(w453) -> ("Modified Config"=w451:T2, "Loaded Config"=w452:T2)
      "Config Out" <- w451
      n262 = Not Equal?(x=w451, y=w452) -> (x != y?=→"Changes?":bool)
    }
  }
